vi "ConveyorBeltLoad.vi"(0 "Barcode":string) -> ()   [LabVIEW 2014]
uses:
  axxon_Gold.vi
panel:
  in  "Com2":T1
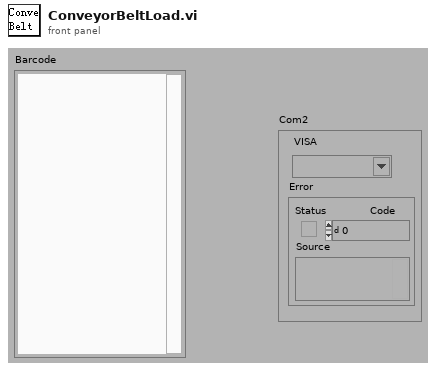
[diagram p1: front panel]
types:
  T1 = cluster{"VISA resource name out":refnum<visa-resource-name>, "error out":errorcluster}
  T2 = typedef "MoveSpeed.ctl" = cluster{"Speed of in board":dbl, "Acc of in board motor":dbl, "Stroke of in board motor":dbl, "Speed of adjusting width motor":dbl, "Acc of adjusting width motor":dbl, "Stroke of adjusting width motor":dbl, "Speed of motor running":dbl, "Acc of motor running":dbl, "Speed of out board":dbl, "Standby Motor Velocity":dbl, "Standby Motor Acceleration:":dbl, "Speed of reflowing motor":dbl, "Speed of reflowing Track Adjusting":dbl, "Acc of reflowing adjusting ":dbl, "Acc of reflowing motor":dbl, "Standby Motor delay":dbl}
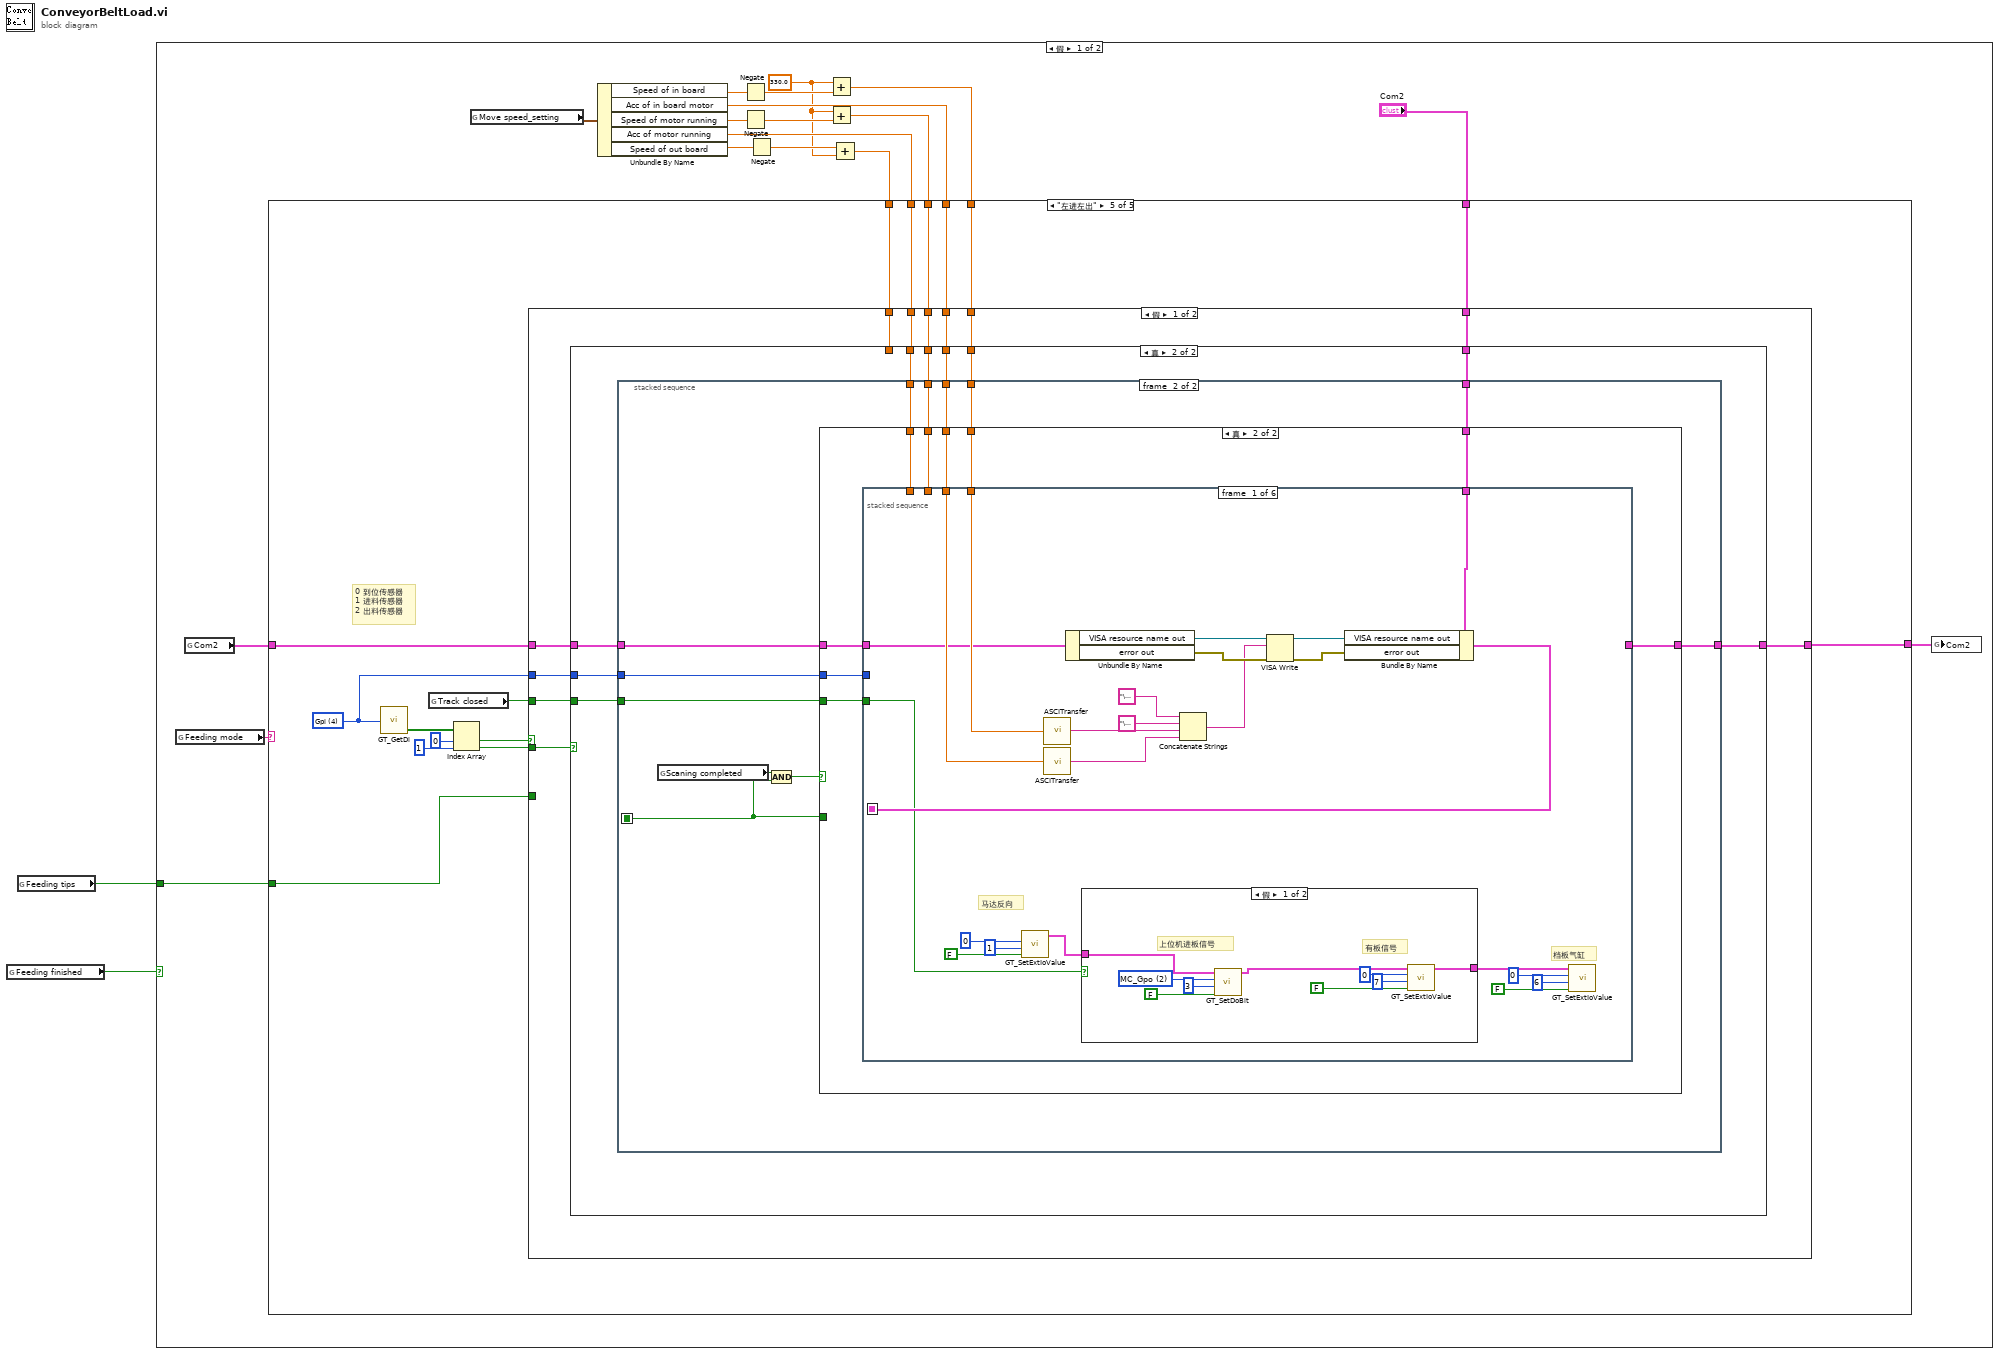
[diagram p0: block diagram]
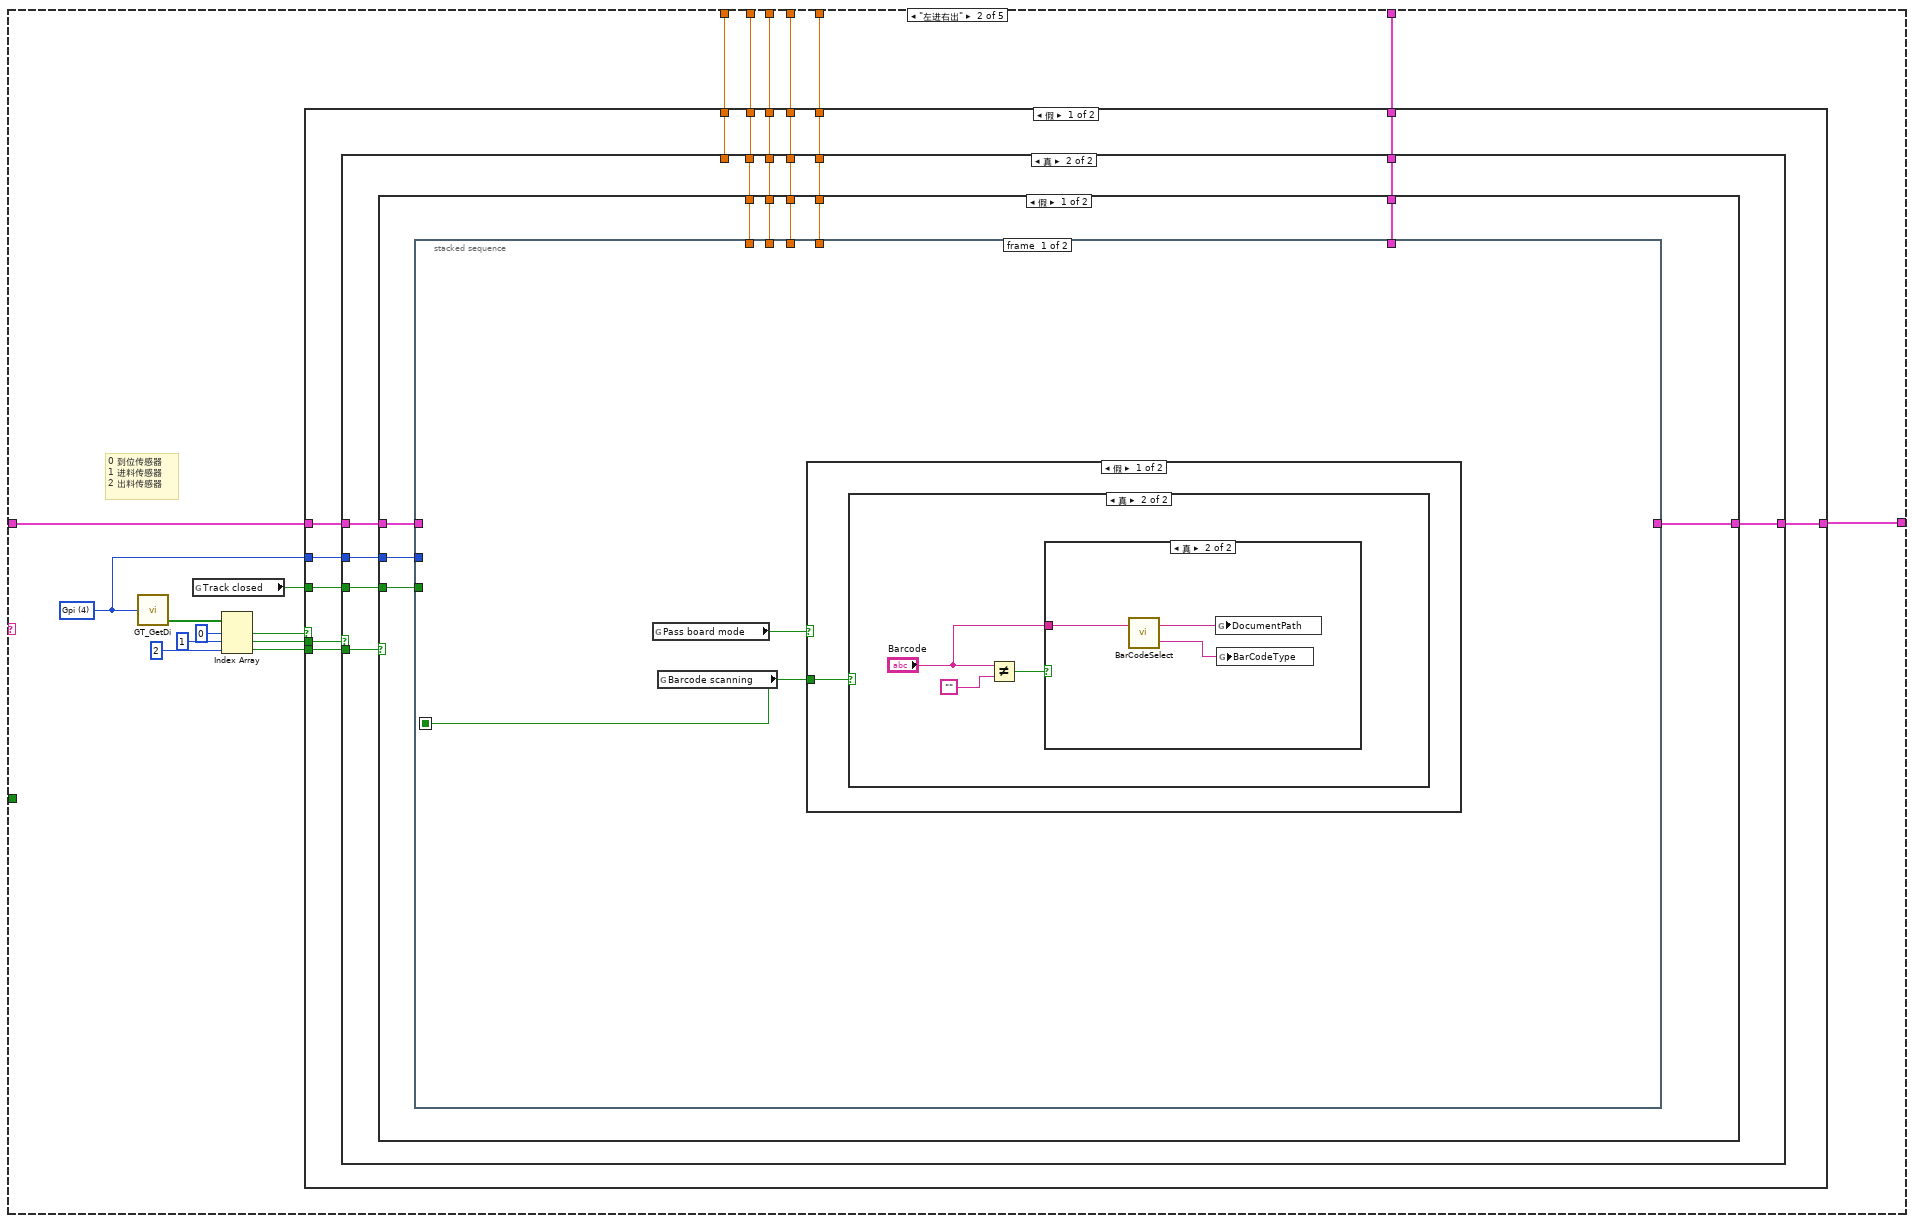
[diagram p3: hidden frame]
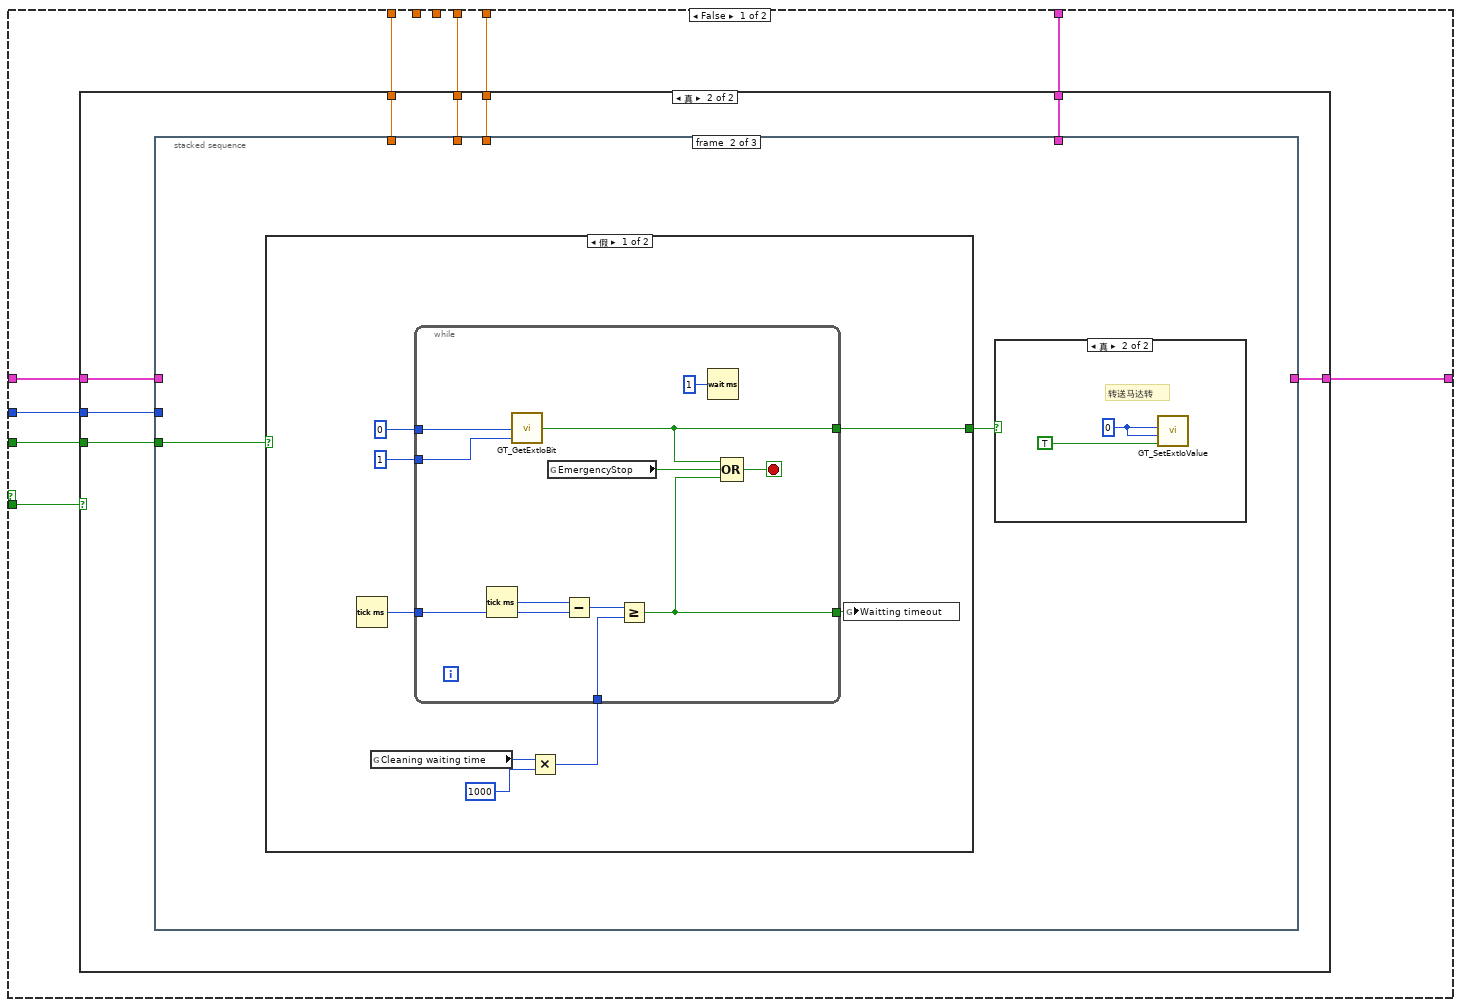
[diagram p4: hidden frame]
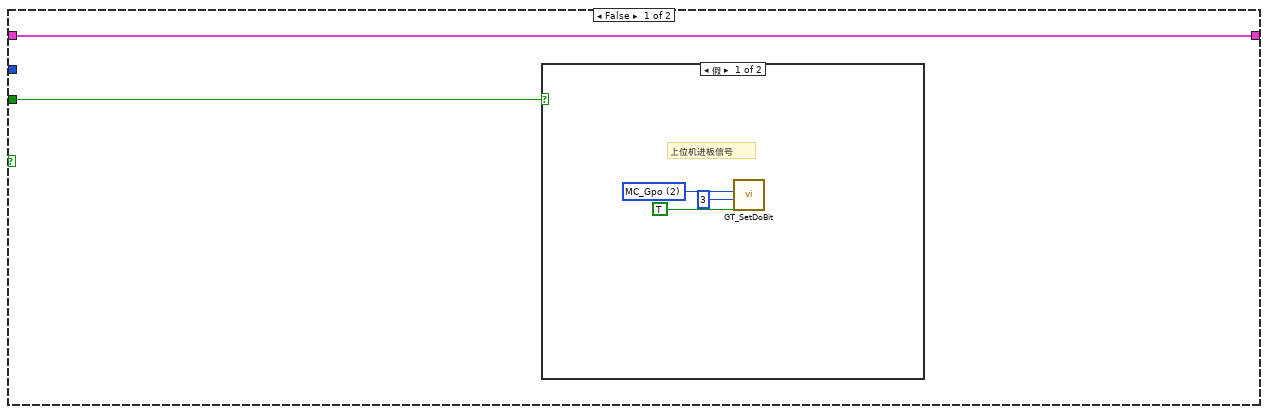
[diagram p5: hidden frame]
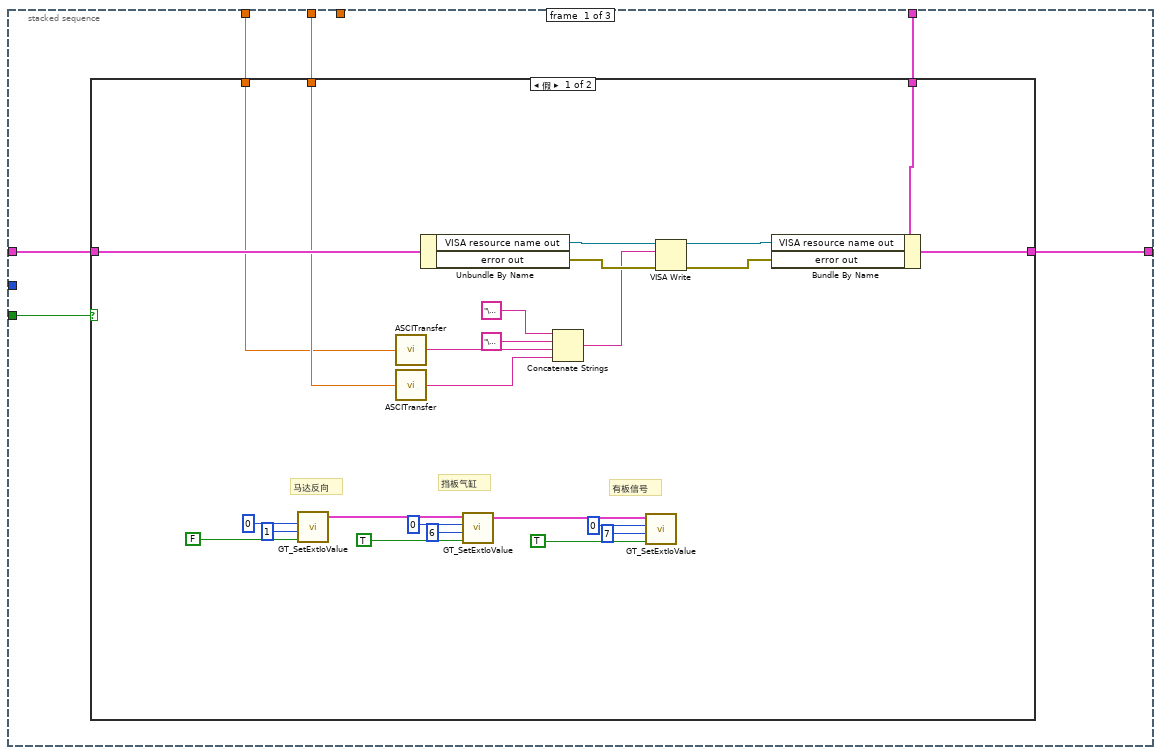
[diagram p7: hidden frame]
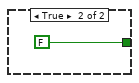
[diagram p10: hidden frame]
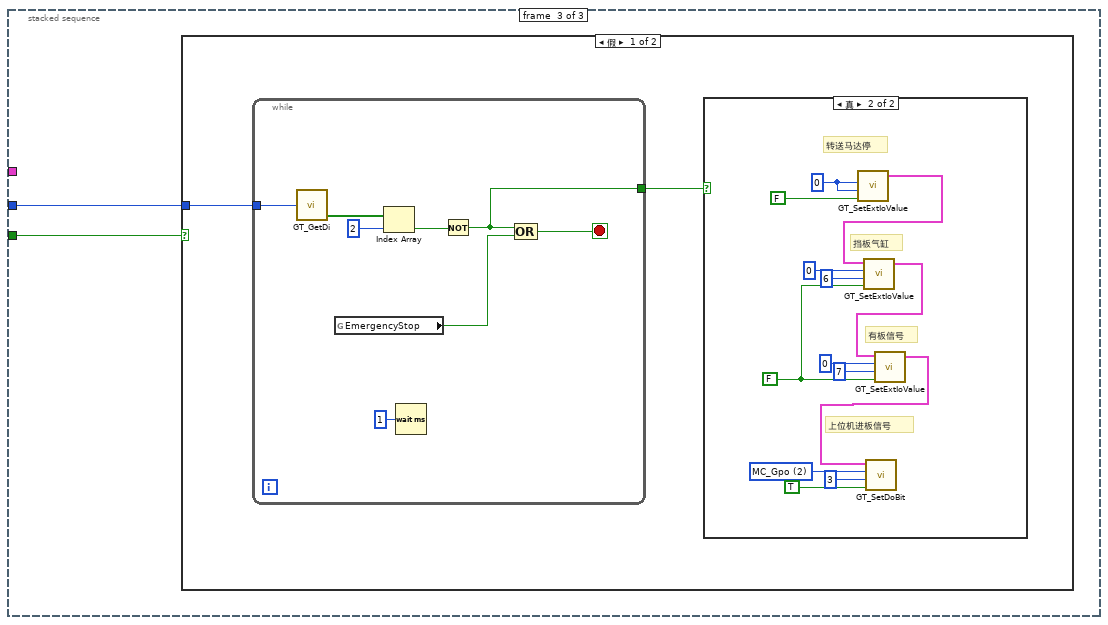
[diagram p11: hidden frame]
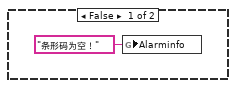
[diagram p15: hidden frame]
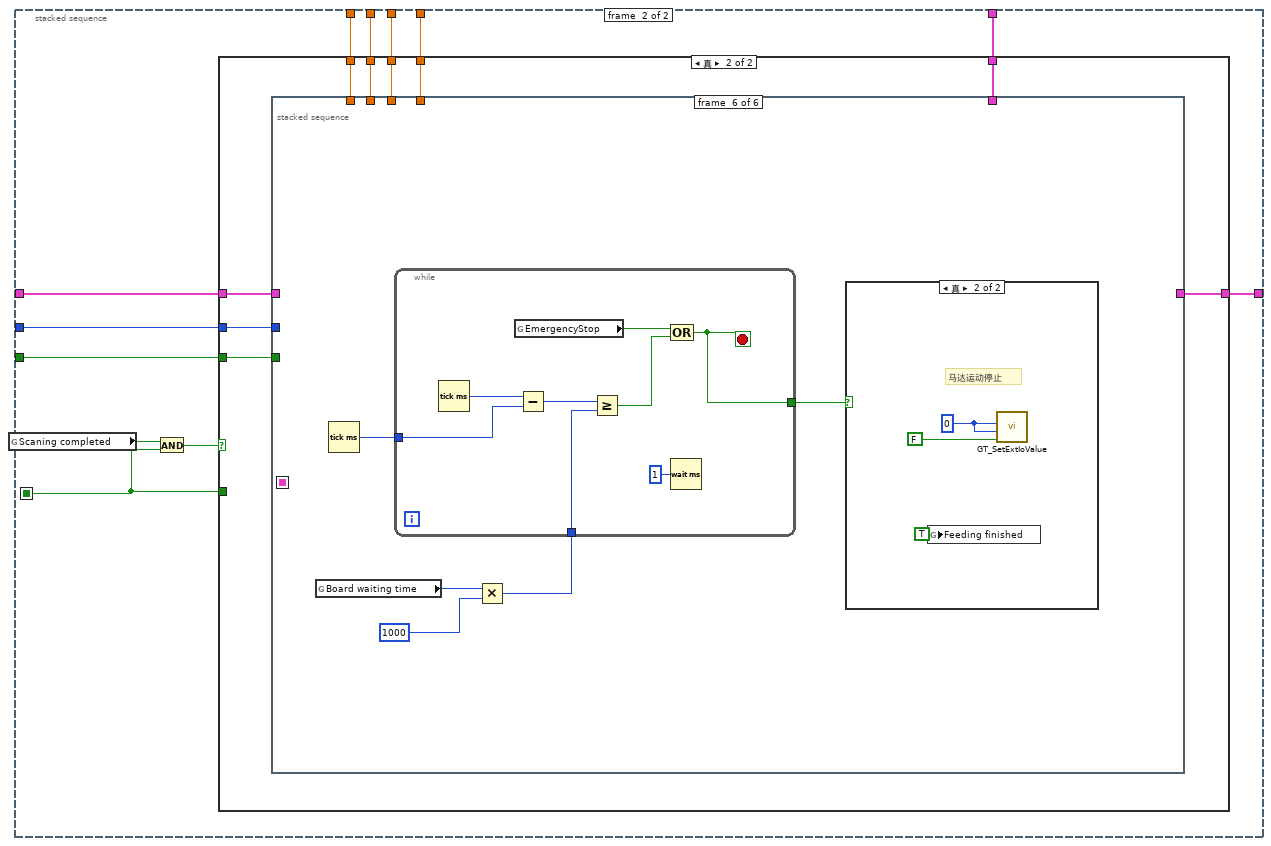
[diagram p17: hidden frame]
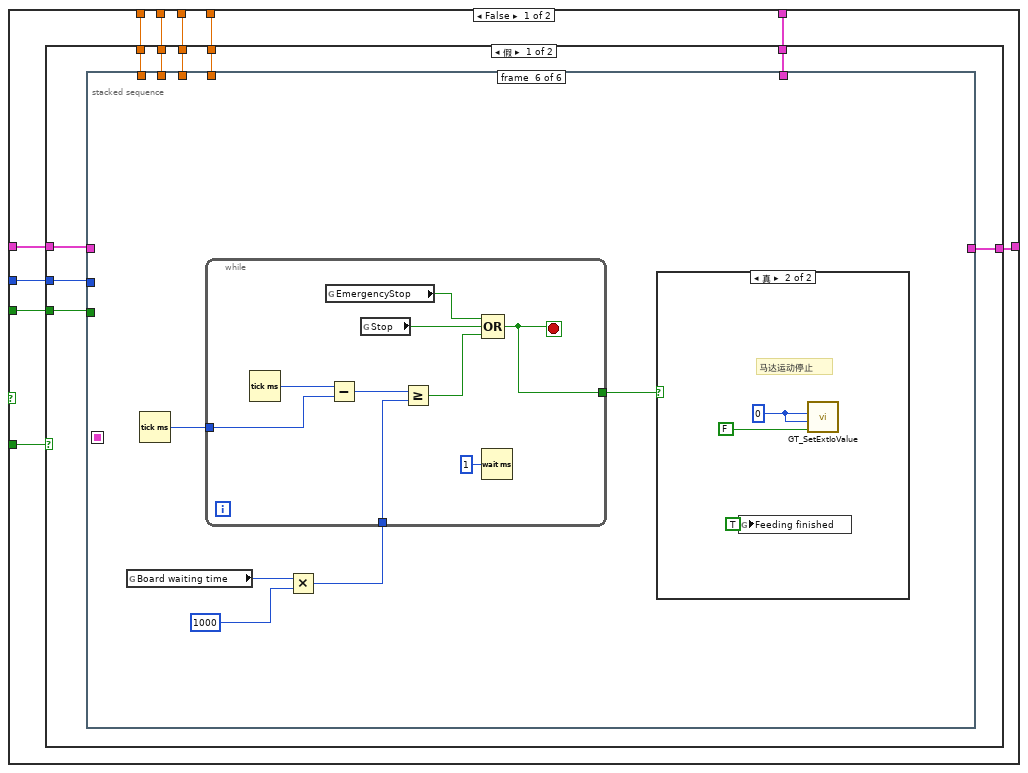
[diagram p18: hidden frame]
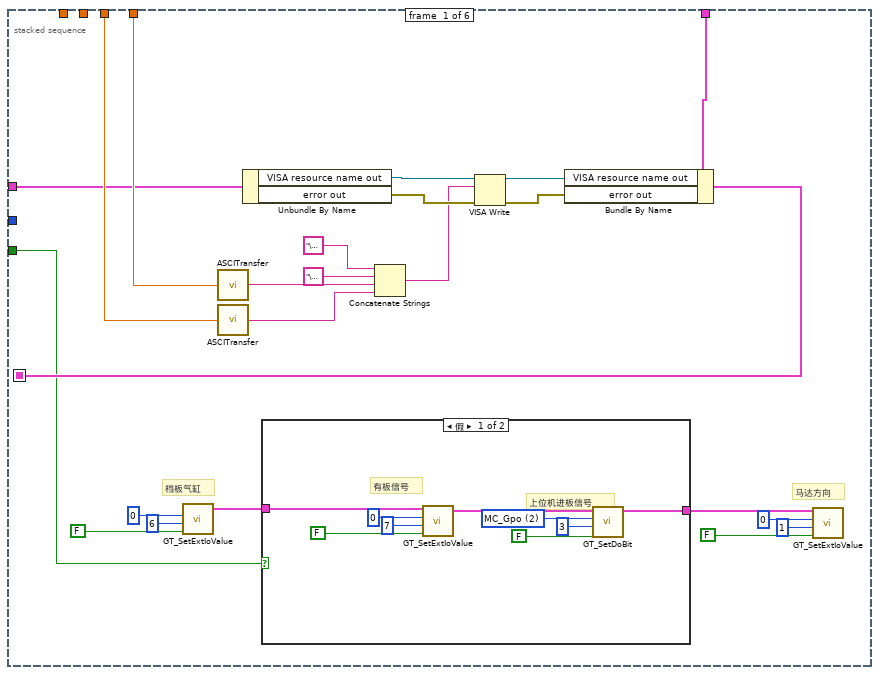
[diagram p19: hidden frame]
diagram:
  n1 = global read "axxon_Gold.vi" "Feeding finished"() -> (w2:bool)
  n2 = global read "axxon_Gold.vi" "Feeding tips"() -> (w1:bool)
  n3 = case shown="假" w2 {
    tunnel: w1 -> [w3 _]
    frame False {
      w7 = 330.0 ("x")
      n4 = global read "axxon_Gold.vi" "Feeding mode"() -> (w5:string)
      n5 = global read "axxon_Gold.vi" "Com2"() -> (w4:T1)
      n6 = global read "axxon_Gold.vi" "Move speed_setting"() -> (w20:T2)
      n7 = Unbundle By Name(w20) -> ("Speed of in board"=w19:dbl, "Acc of in board motor"=w18:dbl, "Speed of motor running"=w15:dbl, "Acc of motor running"=w14:dbl, "Speed of out board"=w9:dbl)
      n8 = Negate(x=w19) -> (-x=w13:dbl)
      n9 = Negate(x=w15) -> (-x=w11:dbl)
      n10 = Negate(x=w9) -> (-x=w8:dbl)
      n11 = Add(x=w7, y=w13) -> (x+y=w12:dbl)
      n12 = Add(x=w7, y=w11) -> (x+y=w10:dbl)
      n13 = Add(x=w8, y=w7) -> (x+y=w6:dbl)
      n14 = case shown="\"左进左出\"" w5 {
        tunnel: w18 -> [_ w31 w535 w1028 w1411]
        tunnel: "Com2" -> [_ w30 w534 w1027 w1410]
        tunnel: [w21 w29 w533 w1026 w1409] -> w16
        tunnel: w14 -> [_ w27 w531 w1024 w1407]
        tunnel: w12 -> [_ w25 w529 w1022 w1405]
        tunnel: w10 -> [_ w24 w528 w1021 w1404]
        tunnel: w6 -> [_ w23 w527 w1020 w1403]
        tunnel: w4 -> [w21 w22 w526 w1019 w1402]
        tunnel: w3 -> [_ _ _ w1018 w1401]
        frame Default {
        }
        frame "左进右出" {
          w28 = i16 4 items=["Limit_Positive", "Limit_Negative", "Alarm", "Home", "Gpi", "arrive"] ("diType in")
          # "0 到位传感器\n1 进料传感器\n2 出料传感器"
          n15 = call "GT_GetDi.vi"("diType in"=w28) -> ("IOOut"=w38:bool[])  [unwired: 2 in, 2 out]
          n16 = global read "axxon_Gold.vi" "Track closed"() -> (w26:bool)
          n17 = Index Array(array=w38, index #1=0 ("索引"), index #2=1 ("索引"), index #3=2 ("索引")) -> (element #1=w34:bool, element #2=w33:bool, element #3=w32:bool)
          n18 = case shown="假" w34 {
            tunnel: w33 -> [w50 _]
            tunnel: w32 -> [w49 _]
            tunnel: w25 -> [w48 w408]
            tunnel: w31 -> [w47 w407]
            tunnel: w30 -> [w46 w404]
            tunnel: w22 -> [w45 w406]
            tunnel: [w44 w405] -> w29
            tunnel: w28 -> [w43 w403]
            tunnel: w24 -> [w42 _]
            tunnel: w27 -> [w41 _]
            tunnel: w26 -> [w40 w402]
            tunnel: w23 -> [w39 w401]
            frame False {
              n19 = case shown="真" w50 {
                tunnel: w49 -> [w59 w163]
                tunnel: w48 -> [w55 w162]
                tunnel: w47 -> [w54 w161]
                tunnel: w46 -> [w56 w160]
                tunnel: w45 -> [w58 w159]
                tunnel: [w57 w158] -> w44
                tunnel: w43 -> [w53 w157]
                tunnel: w42 -> [_ w156]
                tunnel: w41 -> [_ w155]
                tunnel: w40 -> [w52 w154]
                tunnel: w39 -> [w51 _]
                frame False {
                  n20 = case shown="真" w59 {
                    tunnel: w58 -> [w61 w72]
                    tunnel: [w61 w71] -> w57
                    tunnel: w56 -> [_ w70]
                    tunnel: w55 -> [_ w69]
                    tunnel: w54 -> [_ w68]
                    tunnel: w53 -> [_ w67]
                    tunnel: w52 -> [w60 w66]
                    tunnel: w51 -> [_ w65]
                    frame False {
                      n21 = case shown="假" w60 {
                        frame False {
                          w64 = i16 2 items=["MC_Enable", "MC_Clear", "MC_Gpo"] ("doType")
                          # "上位机进板信号"
                          n22 = call "GT_SetDoBit.vi"("Value"=TRUE, "doIndex"=i16 3, "doType"=w64) -> ()  [unwired: 8 in, 1 out]
                        }
                        frame True {
                        }
                      }
                    }
                    frame True {
                      n23 = stacked-sequence {
                        tunnel: w72 -> [w78 _ _]
                        tunnel: [w77 _ _] -> w71
                        tunnel: w70 -> [w76 _ _]
                        tunnel: w69 -> [_ _ _]
                        tunnel: w68 -> [w75 _ _]
                        tunnel: w67 -> [_ _ w130]
                        tunnel: w66 -> [w73 w106 w129]
                        tunnel: w65 -> [w74 _ _]
                        frame #0 {
                          n24 = case shown="假" w73 {
                            tunnel: w78 -> [w94 w104]
                            tunnel: [w93 w104] -> w77
                            tunnel: w76 -> [w92 _]
                            tunnel: w75 -> [w91 _]
                            tunnel: w74 -> [w90 _]
                            frame False {
                              # "马达反向"
                              # "挡板气缸"
                              # "有板信号"
                              n25 = call "GT_SetExtIoValue.vi"("Value"=FALSE, "index"=1, "mdl"=0) -> ("rtn_Out"=w79:cluster{"rtn":i16, "Func":string})  [unwired: 3 in]
                              n26 = call "ASCITransfer.vi"("Input"=w90) -> ("Output"=w99:string)
                              n27 = call "ASCITransfer.vi"("Input"=w91) -> ("Output"=w98:string)
                              n28 = Unbundle By Name(w94) -> ("VISA resource name out"=w103:refnum<visa-resource-name>, "error out"=w102:errorcluster)
                              n29 = call "GT_SetExtIoValue.vi"("Value"=TRUE, "index"=6, "mdl"=0, "rtn_In"=w79) -> ("rtn_Out"=w83:cluster{"rtn":i16, "Func":string})  [unwired: 2 in]
                              n30 = Concatenate Strings("\u001f" ("字符串"), "\u0000" ("字符串"), w99, w98) -> (w97:string)
                              n31 = call "GT_SetExtIoValue.vi"("Value"=TRUE, "index"=7, "mdl"=0, "rtn_In"=w83) -> ()  [unwired: 2 in, 1 out]
                              n32 = VISA Write(VISA resource name=w103, write buffer=w97, error in (no error)=w102) -> (VISA resource name out=w96:refnum<visa-resource-name>, error out=w95:errorcluster)  [unwired: 1 out]
                              n33 = Bundle By Name(cluster=w92, "VISA resource name out"=w96, "error out"=w95) -> (w93:T1)
                            }
                            frame True {
                            }
                          }
                        }
                        frame #1 {
                          n34 = case shown="假" w106 {
                            tunnel: [w115 FALSE] -> w105
                            frame False {
                              n35 = Tick Count (ms)() -> (millisecond timer value=w111:u32)
                              n36 = global read "axxon_Gold.vi" "Cleaning waiting time"() -> (w113:i32)
                              n37 = Multiply(x=w113, y=1000) -> (x*y=w110:i32)
                              n38 = while {
                                tunnel: 0 ("mdl") -> [w127]
                                tunnel: [w122] -> w115
                                tunnel: 1 ("Index") -> [w124]
                                tunnel: w111 -> [w120]
                                tunnel: w110 -> [w118]
                                tunnel: [w117] -> w109
                                stop <- w125 stop-if-true
                                n39 = Tick Count (ms)() -> (millisecond timer value=w121:u32)
                                n40 = call "GT_GetExtIoBit.vi"("Index"=w124, "mdl"=w127) -> ("Status"=w122:bool)  [unwired: 2 in, 1 out]
                                n41 = global read "axxon_Gold.vi" "EmergencyStop"() -> (w123:bool)
                                n42 = Subtract(x=w121, y=w120) -> (x-y=w119:u32)
                                n43 = Greater Or Equal?(x=w119, y=w118) -> (x >= y?=w117:bool)
                                n44 = Wait (ms)(milliseconds to wait=u32 1 ("等待时间（毫秒）")) -> ()  [unwired: 1 out]
                                n45 = Compound Arithmetic op=OR(w122, w123, w117) -> (w125:bool)
                              }
                              n46 = global write "axxon_Gold.vi" "Waitting timeout"(w109) -> ()
                            }
                            frame True {
                            }
                          }
                          n47 = case shown="真" w105 {
                            frame False {
                            }
                            frame True {
                              w108 = 0 ("mdl")
                              # "转送马达转"
                              n48 = call "GT_SetExtIoValue.vi"("Value"=TRUE, "index"=w108, "mdl"=w108) -> ()  [unwired: 3 in, 1 out]
                            }
                          }
                        }
                        frame #2 {
                          n49 = case shown="假" w129 {
                            tunnel: w130 -> [w132 _]
                            frame False {
                              n50 = while {
                                tunnel: w132 -> [w153]
                                tunnel: [w146] -> w131
                                stop <- w148 stop-if-true
                                n51 = call "GT_GetDi.vi"("diType in"=w153) -> ("IOOut"=w152:bool[])  [unwired: 2 in, 2 out]
                                n52 = global read "axxon_Gold.vi" "EmergencyStop"() -> (w147:bool)
                                n53 = Index Array(array=w152, index=2 ("索引")) -> (element=w150:bool)
                                n54 = Wait (ms)(milliseconds to wait=u32 1 ("等待时间（毫秒）")) -> ()  [unwired: 1 out]
                                n55 = Not(x=w150) -> (.not. x?=w146:bool)
                                n56 = Compound Arithmetic op=OR(w146, w147) -> (w148:bool)
                              }
                              n57 = case shown="真" w131 {
                                frame False {
                                }
                                frame True {
                                w141 = i16 2 items=["MC_Enable", "MC_Clear", "MC_Gpo"] ("doType")
                                w134 = FALSE ("Value")
                                w145 = 0 ("mdl")
                                # "上位机进板信号"
                                # "有板信号"
                                # "挡板气缸"
                                # "转送马达停"
                                n58 = call "GT_SetExtIoValue.vi"("Value"=FALSE, "index"=w145, "mdl"=w145) -> ("rtn_Out"=w137:cluster{"rtn":i16, "Func":string})  [unwired: 3 in]
                                n59 = call "GT_SetExtIoValue.vi"("Value"=w134, "index"=6, "mdl"=0, "rtn_In"=w137) -> ("rtn_Out"=w133:cluster{"rtn":i16, "Func":string})  [unwired: 2 in]
                                n60 = call "GT_SetExtIoValue.vi"("Value"=w134, "index"=7, "mdl"=0, "rtn_In"=w133) -> ("rtn_Out"=w138:cluster{"rtn":i16, "Func":string})  [unwired: 2 in]
                                n61 = call "GT_SetDoBit.vi"("Value"=TRUE, "doIndex"=i16 3, "doType"=w141, "rtn_In"=w138) -> ()  [unwired: 7 in, 1 out]
                                }
                              }
                            }
                            frame True {
                            }
                          }
                        }
                      }
                    }
                  }
                }
                frame True {
                  n62 = case shown="假" w163 {
                    tunnel: w162 -> [w172 _]
                    tunnel: w161 -> [w171 _]
                    tunnel: w160 -> [w170 _]
                    tunnel: w159 -> [w169 w400]
                    tunnel: [w168 w400] -> w158
                    tunnel: w157 -> [w167 _]
                    tunnel: w156 -> [w166 _]
                    tunnel: w155 -> [w165 _]
                    tunnel: w154 -> [w164 _]
                    frame False {
                      n63 = stacked-sequence {
                        seq-local: [w173 _] -> [_ w183]
                        tunnel: w172 -> [_ w194]
                        tunnel: w171 -> [_ w193]
                        tunnel: w170 -> [_ w192]
                        tunnel: w169 -> [_ w191]
                        tunnel: [_ w190] -> w168
                        tunnel: w167 -> [_ w189]
                        tunnel: w166 -> [_ w188]
                        tunnel: w165 -> [_ w187]
                        tunnel: w164 -> [_ w186]
                        frame #0 {
                          n64 = global read "axxon_Gold.vi" "Pass board mode"() -> (w174:bool)
                          n65 = global read "axxon_Gold.vi" "Barcode scanning"() -> (w173:bool)
                          n66 = case shown="假" w174 {
                            tunnel: w173 -> [w175 _]
                            frame False {
                              n67 = case shown="真" w175 {
                                frame False {
                                }
                                frame True {
                                n68 = Not Equal?(x="Barcode", y="") -> (x != y?=w176:bool)
                                n69 = case shown="真" w176 {
                                tunnel: "Barcode" -> [_ w182]
                                frame False {
                                n70 = global write "axxon_Gold.vi" "Alarminfo"("条形码为空！" ("Alarminfo")) -> ()
                                }
                                frame True {
                                n71 = call "BarCodeSelect.vi"("BarcodeIn"=w182) -> ("ProductTyple"=w181:string, "ProgramPath"=w180:string)  [unwired: 1 in]
                                n72 = global write "axxon_Gold.vi" "DocumentPath"(w180) -> ()
                                n73 = global write "axxon_Gold.vi" "BarCodeType"(w181) -> ()
                                }
                                }
                                }
                              }
                            }
                            frame True {
                            }
                          }
                        }
                        frame #1 {
                          n74 = global read "axxon_Gold.vi" "Scaning completed"() -> (w184:bool)
                          n75 = And(x=w184, y=w183) -> (x .and. y?=w185:bool)
                          n76 = case shown="真" w185 {
                            tunnel: w194 -> [w197 w317]
                            tunnel: w193 -> [w198 w316]
                            tunnel: w192 -> [w196 w315]
                            tunnel: w191 -> [w203 w314]
                            tunnel: [w195 w313] -> w190
                            tunnel: w189 -> [w202 w312]
                            tunnel: w188 -> [w199 w311]
                            tunnel: w187 -> [w200 w310]
                            tunnel: w186 -> [w201 w309]
                            tunnel: w183 -> [w204 _]
                            frame False {
                              n77 = case shown="假" w204 {
                                tunnel: w203 -> [w213 w308]
                                tunnel: w202 -> [w212 _]
                                tunnel: w201 -> [w211 _]
                                tunnel: w200 -> [w210 _]
                                tunnel: w199 -> [w209 _]
                                tunnel: w198 -> [w208 _]
                                tunnel: w197 -> [w207 _]
                                tunnel: w196 -> [w206 _]
                                tunnel: [w205 w308] -> w195
                                frame False {
                                n78 = stacked-sequence {
                                seq-local: [w223 _ _ _ _ _] -> [_ _ _ w286 _ _]
                                tunnel: w207 -> [w232 _ _ _ _ _]
                                tunnel: w208 -> [w230 _ _ _ _ _]
                                tunnel: w206 -> [w227 _ _ w283 _ _]
                                tunnel: w213 -> [w224 _ _ _ _ _]
                                tunnel: [_ _ _ w282 _ _] -> w205
                                tunnel: w212 -> [_ _ w253 _ _ _]
                                tunnel: w209 -> [_ _ _ w277 _ _]
                                tunnel: w210 -> [_ _ _ w276 _ _]
                                tunnel: w211 -> [w222 _ _ _ _ _]
                                frame #0 {
                                # "马达方向"
                                # "档板气缸"
                                n79 = call "GT_SetExtIoValue.vi"("Value"=FALSE, "index"=6, "mdl"=0) -> ("rtn_Out"=w218:cluster{"rtn":i16, "Func":string})  [unwired: 3 in]
                                n80 = call "ASCITransfer.vi"("Input"=w232) -> ("Output"=w231:string)
                                n81 = call "ASCITransfer.vi"("Input"=w230) -> ("Output"=w229:string)
                                n82 = Unbundle By Name(w224) -> ("VISA resource name out"=w236:refnum<visa-resource-name>, "error out"=w235:errorcluster)
                                n83 = case shown="假" w222 {
                                tunnel: w218 -> [w242 w246]
                                tunnel: [w237 w246] -> w214
                                frame False {
                                w241 = i16 2 items=["MC_Enable", "MC_Clear", "MC_Gpo"] ("doType")
                                # "上位机进板信号"
                                # "有板信号"
                                n84 = call "GT_SetExtIoValue.vi"("Value"=FALSE, "index"=7, "mdl"=0, "rtn_In"=w242) -> ("rtn_Out"=w238:cluster{"rtn":i16, "Func":string})  [unwired: 2 in]
                                n85 = call "GT_SetDoBit.vi"("Value"=FALSE, "doIndex"=i16 3, "doType"=w241, "rtn_In"=w238) -> ("rtn_Out"=w237:cluster{"rtn":i16, "Func":string})  [unwired: 7 in]
                                }
                                frame True {
                                }
                                }
                                n86 = Concatenate Strings("\u001f" ("字符串"), "\u0000" ("字符串"), w231, w229) -> (w228:string)
                                n87 = VISA Write(VISA resource name=w236, write buffer=w228, error in (no error)=w235) -> (VISA resource name out=w226:refnum<visa-resource-name>, error out=w225:errorcluster)  [unwired: 1 out]
                                n88 = Bundle By Name(cluster=w227, "VISA resource name out"=w226, "error out"=w225) -> (w223:T1)
                                n89 = call "GT_SetExtIoValue.vi"("Value"=FALSE, "index"=1, "mdl"=0, "rtn_In"=w214) -> ()  [unwired: 2 in, 1 out]
                                }
                                frame #1 {
                                w249 = 0 ("mdl")
                                # "传送马达运动"
                                n90 = Wait (ms)(milliseconds to wait=u32 100 ("等待时间（毫秒）")) -> ()  [unwired: 1 out]
                                n91 = call "GT_SetExtIoValue.vi"("Value"=TRUE, "index"=w249, "mdl"=w249) -> ()  [unwired: 3 in, 1 out]
                                }
                                frame #2 {
                                n92 = Tick Count (ms)() -> (millisecond timer value=w251:u32)
                                n93 = while {
                                tunnel: w253 -> [w271]
                                tunnel: [w265] -> w252
                                tunnel: w251 -> [w263]
                                tunnel: u32 1500 ("y") -> [w261]
                                stop <- w265 stop-if-true
                                # "到位检测"
                                n94 = Tick Count (ms)() -> (millisecond timer value=w264:u32)
                                n95 = call "GT_GetDi.vi"("diType in"=w271) -> ("IOOut"=w270:bool[])  [unwired: 2 in, 2 out]
                                n96 = Wait (ms)(milliseconds to wait=u32 1 ("等待时间（毫秒）")) -> ()  [unwired: 1 out]
                                n97 = global read "axxon_Gold.vi" "EmergencyStop"() -> (w266:bool)
                                n98 = global read "axxon_Gold.vi" "Stop"() -> (w268:bool)
                                n99 = Subtract(x=w264, y=w263) -> (x-y=w262:u32)
                                n100 = Index Array(array=w270, index=0 ("索引")) -> (element=w260:bool)
                                n101 = Greater Or Equal?(x=w262, y=w261) -> (x >= y?=w259:bool)
                                n102 = case shown="假" w260 {
                                tunnel: w259 -> [w272 _]
                                frame False {
                                n103 = case shown="真" w272 {
                                frame False {
                                }
                                frame True {
                                w274 = 0 ("mdl")
                                n104 = call "GT_SetExtIoValue.vi"("Value"=TRUE, "index"=w274, "mdl"=w274) -> ()  [unwired: 3 in, 1 out]
                                }
                                }
                                }
                                frame True {
                                }
                                }
                                n105 = Compound Arithmetic op=OR(w260, w268, w266) -> (w265:bool)
                                }
                                n106 = case shown="真" w252 {
                                frame False {
                                }
                                frame True {
                                w254 = FALSE ("Value")
                                w258 = 0 ("mdl")
                                # "档板气缸"
                                # "传送马达停止"
                                n107 = call "GT_SetExtIoValue.vi"("Value"=w254, "index"=6, "mdl"=0) -> ("rtn_Out"=w255:cluster{"rtn":i16, "Func":string})  [unwired: 3 in]
                                n108 = call "GT_SetExtIoValue.vi"("Value"=w254, "index"=w258, "mdl"=w258, "rtn_In"=w255) -> ()  [unwired: 2 in, 1 out]
                                }
                                }
                                }
                                frame #3 {
                                n109 = call "ASCITransfer.vi"("Input"=w277) -> ("Output"=w279:string)
                                n110 = call "ASCITransfer.vi"("Input"=w276) -> ("Output"=w278:string)
                                n111 = Unbundle By Name(w286) -> ("VISA resource name out"=w288:refnum<visa-resource-name>, "error out"=w285:errorcluster)
                                n112 = Concatenate Strings("\u001f" ("字符串"), "\u0000" ("字符串"), w279, w278) -> (w275:string)
                                n113 = VISA Write(VISA resource name=w288, write buffer=w275, error in (no error)=w285) -> (VISA resource name out=w287:refnum<visa-resource-name>, error out=w284:errorcluster)  [unwired: 1 out]
                                n114 = Bundle By Name(cluster=w283, "VISA resource name out"=w287, "error out"=w284) -> (w282:T1)
                                }
                                frame #4 {
                                w290 = 0 ("mdl")
                                # "传送马达动"
                                n115 = call "GT_SetExtIoValue.vi"("Value"=TRUE, "index"=w290, "mdl"=w290) -> ()  [unwired: 3 in, 1 out]
                                }
                                frame #5 {
                                n116 = global read "axxon_Gold.vi" "Board waiting time"() -> (w294:u32)
                                n117 = Tick Count (ms)() -> (millisecond timer value=w295:u32)
                                n118 = Multiply(x=w294, y=u32 1000) -> (x*y=w292:u32)
                                n119 = while {
                                tunnel: w295 -> [w306]
                                tunnel: w292 -> [w304]
                                tunnel: [w300] -> w291
                                stop <- w300 stop-if-true
                                n120 = Tick Count (ms)() -> (millisecond timer value=w307:u32)
                                n121 = global read "axxon_Gold.vi" "EmergencyStop"() -> (w299:bool)
                                n122 = Subtract(x=w307, y=w306) -> (x-y=w305:u32)
                                n123 = global read "axxon_Gold.vi" "Stop"() -> (w303:bool)
                                n124 = Greater Or Equal?(x=w305, y=w304) -> (x >= y?=w302:bool)
                                n125 = Compound Arithmetic op=OR(w299, w303, w302) -> (w300:bool)
                                n126 = Wait (ms)(milliseconds to wait=u32 1 ("等待时间（毫秒）")) -> ()  [unwired: 1 out]
                                }
                                n127 = case shown="真" w291 {
                                frame False {
                                }
                                frame True {
                                w298 = 0 ("mdl")
                                # "马达运动停止"
                                n128 = global write "axxon_Gold.vi" "Feeding finished"(TRUE ("进板完成")) -> ()
                                n129 = call "GT_SetExtIoValue.vi"("Value"=FALSE, "index"=w298, "mdl"=w298) -> ()  [unwired: 3 in, 1 out]
                                }
                                }
                                }
                                }
                                }
                                frame True {
                                }
                              }
                            }
                            frame True {
                              n130 = stacked-sequence {
                                seq-local: [w327 _ _ _ _ _] -> [_ _ _ w379 _ _]
                                tunnel: w317 -> [w336 _ _ _ _ _]
                                tunnel: w316 -> [w334 _ _ _ _ _]
                                tunnel: w315 -> [w331 _ _ w376 _ _]
                                tunnel: w314 -> [w328 _ _ _ _ _]
                                tunnel: [_ _ _ w375 _ _] -> w313
                                tunnel: w312 -> [_ _ w354 _ _ _]
                                tunnel: w311 -> [_ _ _ w370 _ _]
                                tunnel: w310 -> [_ _ _ w369 _ _]
                                tunnel: w309 -> [w326 _ _ _ _ _]
                                frame #0 {
                                # "马达反向"
                                # "档板气缸"
                                n131 = call "GT_SetExtIoValue.vi"("Value"=FALSE, "index"=1, "mdl"=0) -> ("rtn_Out"=w318:cluster{"rtn":i16, "Func":string})  [unwired: 3 in]
                                n132 = call "ASCITransfer.vi"("Input"=w336) -> ("Output"=w335:string)
                                n133 = call "ASCITransfer.vi"("Input"=w334) -> ("Output"=w333:string)
                                n134 = Unbundle By Name(w328) -> ("VISA resource name out"=w340:refnum<visa-resource-name>, "error out"=w339:errorcluster)
                                n135 = case shown="假" w326 {
                                tunnel: w318 -> [w343 w350]
                                tunnel: [w341 w350] -> w322
                                frame False {
                                w349 = i16 2 items=["MC_Enable", "MC_Clear", "MC_Gpo"] ("doType")
                                # "有板信号"
                                # "上位机进板信号"
                                n136 = call "GT_SetDoBit.vi"("Value"=FALSE, "doIndex"=i16 3, "doType"=w349, "rtn_In"=w343) -> ("rtn_Out"=w342:cluster{"rtn":i16, "Func":string})  [unwired: 7 in]
                                n137 = call "GT_SetExtIoValue.vi"("Value"=FALSE, "index"=7, "mdl"=0, "rtn_In"=w342) -> ("rtn_Out"=w341:cluster{"rtn":i16, "Func":string})  [unwired: 2 in]
                                }
                                frame True {
                                }
                                }
                                n138 = Concatenate Strings("\u001f" ("字符串"), "\u0000" ("字符串"), w335, w333) -> (w332:string)
                                n139 = VISA Write(VISA resource name=w340, write buffer=w332, error in (no error)=w339) -> (VISA resource name out=w330:refnum<visa-resource-name>, error out=w329:errorcluster)  [unwired: 1 out]
                                n140 = Bundle By Name(cluster=w331, "VISA resource name out"=w330, "error out"=w329) -> (w327:T1)
                                n141 = call "GT_SetExtIoValue.vi"("Value"=FALSE, "index"=6, "mdl"=0, "rtn_In"=w322) -> ()  [unwired: 2 in, 1 out]
                                }
                                frame #1 {
                                w352 = 0 ("mdl")
                                # "传送马达运动"
                                n142 = call "GT_SetExtIoValue.vi"("Value"=TRUE, "index"=w352, "mdl"=w352) -> ()  [unwired: 3 in, 1 out]
                                }
                                frame #2 {
                                n143 = while {
                                tunnel: w354 -> [w367]
                                tunnel: [w362] -> w353
                                stop <- w362 stop-if-true
                                # "到位检测"
                                n144 = call "GT_GetDi.vi"("diType in"=w367) -> ("IOOut"=w366:bool[])  [unwired: 2 in, 2 out]
                                n145 = Wait (ms)(milliseconds to wait=u32 1 ("等待时间（毫秒）")) -> ()  [unwired: 1 out]
                                n146 = global read "axxon_Gold.vi" "EmergencyStop"() -> (w361:bool)
                                n147 = Index Array(array=w366, index=0 ("索引")) -> (element=w364:bool)
                                n148 = Compound Arithmetic op=OR(w364, w361) -> (w362:bool)
                                }
                                n149 = case shown="真" w353 {
                                frame False {
                                }
                                frame True {
                                w360 = 0 ("mdl")
                                # "档板气缸"
                                # "传送马达停止"
                                n150 = call "GT_SetExtIoValue.vi"("Value"=FALSE, "index"=6, "mdl"=0) -> ("rtn_Out"=w355:cluster{"rtn":i16, "Func":string})  [unwired: 3 in]
                                n151 = call "GT_SetExtIoValue.vi"("Value"=FALSE, "index"=w360, "mdl"=w360, "rtn_In"=w355) -> ()  [unwired: 2 in, 1 out]
                                }
                                }
                                }
                                frame #3 {
                                n152 = call "ASCITransfer.vi"("Input"=w370) -> ("Output"=w372:string)
                                n153 = call "ASCITransfer.vi"("Input"=w369) -> ("Output"=w371:string)
                                n154 = Unbundle By Name(w379) -> ("VISA resource name out"=w381:refnum<visa-resource-name>, "error out"=w378:errorcluster)
                                n155 = Concatenate Strings("\u001f" ("字符串"), "\u0000" ("字符串"), w372, w371) -> (w368:string)
                                n156 = VISA Write(VISA resource name=w381, write buffer=w368, error in (no error)=w378) -> (VISA resource name out=w380:refnum<visa-resource-name>, error out=w377:errorcluster)  [unwired: 1 out]
                                n157 = Bundle By Name(cluster=w376, "VISA resource name out"=w380, "error out"=w377) -> (w375:T1)
                                }
                                frame #4 {
                                w383 = 0 ("mdl")
                                # "传送马达动"
                                n158 = call "GT_SetExtIoValue.vi"("Value"=TRUE, "index"=w383, "mdl"=w383) -> ()  [unwired: 3 in, 1 out]
                                }
                                frame #5 {
                                n159 = global read "axxon_Gold.vi" "Board waiting time"() -> (w387:u32)
                                n160 = Tick Count (ms)() -> (millisecond timer value=w388:u32)
                                n161 = Multiply(x=w387, y=u32 1000) -> (x*y=w385:u32)
                                n162 = while {
                                tunnel: w388 -> [w398]
                                tunnel: w385 -> [w396]
                                tunnel: [w393] -> w384
                                stop <- w393 stop-if-true
                                n163 = Tick Count (ms)() -> (millisecond timer value=w399:u32)
                                n164 = global read "axxon_Gold.vi" "EmergencyStop"() -> (w392:bool)
                                n165 = Subtract(x=w399, y=w398) -> (x-y=w397:u32)
                                n166 = Greater Or Equal?(x=w397, y=w396) -> (x >= y?=w395:bool)
                                n167 = Compound Arithmetic op=OR(w392, w395) -> (w393:bool)
                                n168 = Wait (ms)(milliseconds to wait=u32 1 ("等待时间（毫秒）")) -> ()  [unwired: 1 out]
                                }
                                n169 = case shown="真" w384 {
                                frame False {
                                }
                                frame True {
                                w391 = 0 ("mdl")
                                # "马达运动停止"
                                n170 = global write "axxon_Gold.vi" "Feeding finished"(TRUE ("进板完成")) -> ()
                                n171 = call "GT_SetExtIoValue.vi"("Value"=FALSE, "index"=w391, "mdl"=w391) -> ()  [unwired: 3 in, 1 out]
                                }
                                }
                                }
                              }
                            }
                          }
                        }
                      }
                    }
                    frame True {
                    }
                  }
                }
              }
            }
            frame True {
              n172 = stacked-sequence {
                seq-local: [w412 _ _ _ _ _] -> [_ w434 w442 w445 w469 w497]
                tunnel: w408 -> [_ _ _ _ _ _]
                tunnel: w407 -> [w417 _ _ _ _ _]
                tunnel: w406 -> [w416 _ _ _ _ _]
                tunnel: [w415 _ _ _ _ _] -> w405
                tunnel: w404 -> [w414 _ _ _ _ _]
                tunnel: w403 -> [_ _ _ w447 _ w499]
                tunnel: w402 -> [_ _ _ w446 w470 w498]
                tunnel: w401 -> [w413 _ _ _ _ _]
                frame #0 {
                  n173 = Two Button Dialog(message="轨道上有板，是否继续涂！" ("消息"), 1:"取消" ("F按钮名称（“取消”）"), 2:"确定" ("T按钮名称（“确定”）")) -> (T button?=w412:bool)
                  n174 = case shown="真" w412 {
                    tunnel: w417 -> [w422 _]
                    tunnel: w416 -> [w421 w433]
                    tunnel: [w420 w433] -> w415
                    tunnel: w414 -> [w419 _]
                    tunnel: w413 -> [w418 _]
                    frame False {
                      n175 = call "ASCITransfer.vi"("Input"=w418) -> ("Output"=w427:string)
                      n176 = call "ASCITransfer.vi"("Input"=w422) -> ("Output"=w426:string)
                      n177 = Unbundle By Name(w421) -> ("VISA resource name out"=w431:refnum<visa-resource-name>, "error out"=w430:errorcluster)
                      n178 = Concatenate Strings("\u001f" ("字符串"), "\u0000" ("字符串"), w427, w426) -> (w425:string)
                      n179 = VISA Write(VISA resource name=w431, write buffer=w425, error in (no error)=w430) -> (VISA resource name out=w424:refnum<visa-resource-name>, error out=w423:errorcluster)  [unwired: 1 out]
                      n180 = Bundle By Name(cluster=w419, "VISA resource name out"=w424, "error out"=w423) -> (w420:T1)
                    }
                    frame True {
                      n181 = global write "axxon_Gold.vi" "Feeding finished"(TRUE ("进板完成")) -> ()
                    }
                  }
                }
                frame #1 {
                  n182 = case shown="假" w434 {
                    frame False {
                      # "马达反向"
                      # "挡板气缸"
                      n183 = call "GT_SetExtIoValue.vi"("Value"=TRUE, "index"=6, "mdl"=0) -> ("rtn_Out"=w435:cluster{"rtn":i16, "Func":string})  [unwired: 3 in]
                      n184 = call "GT_SetExtIoValue.vi"("Value"=FALSE, "index"=1, "mdl"=0, "rtn_In"=w435) -> ()  [unwired: 2 in, 1 out]
                    }
                    frame True {
                    }
                  }
                }
                frame #2 {
                  n185 = case shown="假" w442 {
                    frame False {
                      w444 = 0 ("mdl")
                      # "传送马达运动"
                      n186 = call "GT_SetExtIoValue.vi"("Value"=TRUE, "index"=w444, "mdl"=w444) -> ()  [unwired: 3 in, 1 out]
                    }
                    frame True {
                    }
                  }
                }
                frame #3 {
                  n187 = case shown="假" w445 {
                    tunnel: w447 -> [w450 _]
                    tunnel: w446 -> [w448 _]
                    frame False {
                      n188 = while {
                        tunnel: w450 -> [w468]
                        tunnel: [w463] -> w449
                        stop <- w463 stop-if-true
                        n189 = call "GT_GetDi.vi"("diType in"=w468) -> ("IOOut"=w467:bool[])  [unwired: 2 in, 2 out]
                        n190 = global read "axxon_Gold.vi" "EmergencyStop"() -> (w462:bool)
                        n191 = Index Array(array=w467, index=2 ("索引")) -> (element=w465:bool)
                        n192 = Compound Arithmetic op=OR(w465, w462) -> (w463:bool)
                        n193 = Wait (ms)(milliseconds to wait=u32 1 ("等待时间（毫秒）")) -> ()  [unwired: 1 out]
                      }
                      n194 = case shown="真" w449 {
                        tunnel: w448 -> [_ w451]
                        frame False {
                        }
                        frame True {
                          n195 = stacked-sequence {
                            tunnel: w451 -> [w452 _]
                            frame #0 {
                              n196 = case shown="真" w452 {
                                frame False {
                                }
                                frame True {
                                n197 = global read "axxon_Gold.vi" "Discharge waiting time"() -> (w455:dbl)
                                n198 = Multiply(x=w455, y=1000.0) -> (x*y=w453:dbl)
                                n199 = Wait (ms)(milliseconds to wait=w453) -> ()  [unwired: 1 out]
                                }
                              }
                            }
                            frame #1 {
                              w461 = 0 ("mdl")
                              # "挡板气缸"
                              # "传送马达停止"
                              n200 = call "GT_SetExtIoValue.vi"("Value"=FALSE, "index"=w461, "mdl"=w461) -> ("rtn_Out"=w456:cluster{"rtn":i16, "Func":string})  [unwired: 3 in]
                              n201 = call "GT_SetExtIoValue.vi"("Value"=FALSE, "index"=6, "mdl"=0, "rtn_In"=w456) -> ()  [unwired: 2 in, 1 out]
                            }
                          }
                        }
                      }
                    }
                    frame True {
                    }
                  }
                }
                frame #4 {
                  n202 = case shown="假" w469 {
                    tunnel: w470 -> [w474 _]
                    frame False {
                      n203 = case shown="假" w474 {
                        tunnel: 0 ("mdl") -> [w484 _]
                        tunnel: [w483 FALSE] -> w472
                        tunnel: 1 ("Index") -> [w482 _]
                        frame False {
                          n204 = global read "axxon_Gold.vi" "Cleaning waiting time"() -> (w481:i32)
                          n205 = Tick Count (ms)() -> (millisecond timer value=w479:u32)
                          n206 = Multiply(x=w481, y=1000) -> (x*y=w478:i32)
                          n207 = while {
                            tunnel: w484 -> [w495]
                            tunnel: [w490] -> w483
                            tunnel: w482 -> [w492]
                            tunnel: w479 -> [w488]
                            tunnel: w478 -> [w486]
                            tunnel: [w485] -> w477
                            stop <- w493 stop-if-true
                            # "下位机进板信号"
                            n208 = Tick Count (ms)() -> (millisecond timer value=w489:u32)
                            n209 = call "GT_GetExtIoBit.vi"("Index"=w492, "mdl"=w495) -> ("Status"=w490:bool)  [unwired: 2 in, 1 out]
                            n210 = global read "axxon_Gold.vi" "EmergencyStop"() -> (w491:bool)
                            n211 = Subtract(x=w489, y=w488) -> (x-y=w487:u32)
                            n212 = Greater Or Equal?(x=w487, y=w486) -> (x >= y?=w485:bool)
                            n213 = Compound Arithmetic op=OR(w490, w491, w485) -> (w493:bool)
                            n214 = Wait (ms)(milliseconds to wait=u32 1 ("等待时间（毫秒）")) -> ()  [unwired: 1 out]
                          }
                          n215 = global write "axxon_Gold.vi" "Waitting timeout"(w477) -> ()
                        }
                        frame True {
                          # "离线模式"
                        }
                      }
                      n216 = case shown="假" w472 {
                        frame False {
                        }
                        frame True {
                          w476 = 0 ("mdl")
                          # "传送马达动"
                          n217 = call "GT_SetExtIoValue.vi"("Value"=TRUE, "index"=w476, "mdl"=w476) -> ()  [unwired: 3 in, 1 out]
                        }
                      }
                    }
                    frame True {
                    }
                  }
                }
                frame #5 {
                  n218 = case shown="假" w497 {
                    tunnel: w499 -> [w501 _]
                    tunnel: w498 -> [w500 _]
                    frame False {
                      n219 = case shown="假" w500 {
                        tunnel: w501 -> [w503 _]
                        frame False {
                          n220 = while {
                            tunnel: w503 -> [w525]
                            tunnel: [w520] -> w502
                            stop <- w520 stop-if-true
                            n221 = call "GT_GetDi.vi"("diType in"=w525) -> ("IOOut"=w524:bool[])  [unwired: 2 in, 2 out]
                            n222 = global read "axxon_Gold.vi" "EmergencyStop"() -> (w518:bool)
                            n223 = Index Array(array=w524, index=2 ("索引")) -> (element=w522:bool)
                            n224 = Not(x=w522) -> (.not. x?=w521:bool)
                            n225 = Wait (ms)(milliseconds to wait=u32 1 ("等待时间（毫秒）")) -> ()  [unwired: 1 out]
                            n226 = Compound Arithmetic op=OR(w521, w518) -> (w520:bool)
                          }
                          n227 = case shown="真" w502 {
                            frame False {
                            }
                            frame True {
                              w510 = i16 2 items=["MC_Enable", "MC_Clear", "MC_Gpo"] ("doType")
                              w517 = 0 ("mdl")
                              # "上位机进板信号"
                              # "有板信号"
                              # "挡板气缸"
                              # "传送马达停"
                              n228 = call "GT_SetExtIoValue.vi"("Value"=FALSE, "index"=w517, "mdl"=w517) -> ("rtn_Out"=w506:cluster{"rtn":i16, "Func":string})  [unwired: 3 in]
                              n229 = call "GT_SetExtIoValue.vi"("Value"=FALSE, "index"=6, "mdl"=0, "rtn_In"=w506) -> ("rtn_Out"=w505:cluster{"rtn":i16, "Func":string})  [unwired: 2 in]
                              n230 = call "GT_SetExtIoValue.vi"("Value"=FALSE, "index"=7, "mdl"=0, "rtn_In"=w505) -> ("rtn_Out"=w504:cluster{"rtn":i16, "Func":string})  [unwired: 2 in]
                              n231 = call "GT_SetDoBit.vi"("Value"=TRUE, "doIndex"=i16 3, "doType"=w510, "rtn_In"=w504) -> ()  [unwired: 7 in, 1 out]
                            }
                          }
                        }
                        frame True {
                        }
                      }
                    }
                    frame True {
                    }
                  }
                }
              }
            }
          }
        }
        frame "右进左出" {
          w532 = i16 4 items=["Limit_Positive", "Limit_Negative", "Alarm", "Home", "Gpi", "arrive"] ("diType in")
          # "0 到位传感器\n1 出料传感器\n2 进料传感器"
          n232 = call "GT_GetDi.vi"("diType in"=w532) -> ("IOOut"=w542:bool[])  [unwired: 2 in, 2 out]
          n233 = global read "axxon_Gold.vi" "Track closed"() -> (w530:bool)
          n234 = Index Array(array=w542, index #1=0 ("索引"), index #2=2 ("索引"), index #3=1 ("索引")) -> (element #1=w538:bool, element #2=w537:bool, element #3=w536:bool)
          n235 = case shown="假" w538 {
            tunnel: w537 -> [w554 _]
            tunnel: w536 -> [w553 _]
            tunnel: w529 -> [w552 w901]
            tunnel: w535 -> [w551 w900]
            tunnel: w534 -> [w550 w897]
            tunnel: w526 -> [w549 w899]
            tunnel: [w548 w898] -> w533
            tunnel: w532 -> [w547 w896]
            tunnel: w528 -> [w546 _]
            tunnel: w531 -> [w545 _]
            tunnel: w530 -> [w544 w895]
            tunnel: w527 -> [w543 w894]
            frame False {
              n236 = case shown="真" w554 {
                tunnel: w553 -> [w563 w667]
                tunnel: w552 -> [w559 w666]
                tunnel: w551 -> [w558 w665]
                tunnel: w550 -> [w560 w664]
                tunnel: w549 -> [w562 w663]
                tunnel: [w561 w662] -> w548
                tunnel: w547 -> [w557 w661]
                tunnel: w546 -> [_ w660]
                tunnel: w545 -> [_ w659]
                tunnel: w544 -> [w556 w658]
                tunnel: w543 -> [w555 _]
                frame False {
                  n237 = case shown="真" w563 {
                    tunnel: w562 -> [w565 w576]
                    tunnel: [w565 w575] -> w561
                    tunnel: w560 -> [_ w574]
                    tunnel: w559 -> [_ w573]
                    tunnel: w558 -> [_ w572]
                    tunnel: w557 -> [_ w571]
                    tunnel: w556 -> [w564 w570]
                    tunnel: w555 -> [_ w569]
                    frame False {
                      n238 = case shown="真" w564 {
                        frame False {
                          w568 = i16 2 items=["MC_Enable", "MC_Clear", "MC_Gpo"] ("doType")
                          # "上位机进板信号"
                          n239 = call "GT_SetDoBit.vi"("Value"=TRUE, "doIndex"=i16 3, "doType"=w568) -> ()  [unwired: 8 in, 1 out]
                        }
                        frame True {
                        }
                      }
                    }
                    frame True {
                      n240 = stacked-sequence {
                        tunnel: w576 -> [w582 _ _]
                        tunnel: [w581 _ _] -> w575
                        tunnel: w574 -> [w580 _ _]
                        tunnel: w573 -> [_ _ _]
                        tunnel: w572 -> [w579 _ _]
                        tunnel: w571 -> [_ _ w634]
                        tunnel: w570 -> [w577 w610 w633]
                        tunnel: w569 -> [w578 _ _]
                        frame #0 {
                          n241 = case shown="真" w577 {
                            tunnel: w582 -> [w598 w608]
                            tunnel: [w597 w608] -> w581
                            tunnel: w580 -> [w596 _]
                            tunnel: w579 -> [w595 _]
                            tunnel: w578 -> [w594 _]
                            frame False {
                              # "马达反向"
                              # "挡板气缸"
                              # "有板信号"
                              n242 = call "ASCITransfer.vi"("Input"=w594) -> ("Output"=w603:string)
                              n243 = call "ASCITransfer.vi"("Input"=w595) -> ("Output"=w602:string)
                              n244 = call "GT_SetExtIoValue.vi"("Value"=TRUE, "index"=1, "mdl"=0) -> ("rtn_Out"=w583:cluster{"rtn":i16, "Func":string})  [unwired: 3 in]
                              n245 = Unbundle By Name(w598) -> ("VISA resource name out"=w607:refnum<visa-resource-name>, "error out"=w606:errorcluster)
                              n246 = Concatenate Strings("\u001f" ("字符串"), "\u0000" ("字符串"), w603, w602) -> (w601:string)
                              n247 = call "GT_SetExtIoValue.vi"("Value"=TRUE, "index"=6, "mdl"=0, "rtn_In"=w583) -> ("rtn_Out"=w587:cluster{"rtn":i16, "Func":string})  [unwired: 2 in]
                              n248 = VISA Write(VISA resource name=w607, write buffer=w601, error in (no error)=w606) -> (VISA resource name out=w600:refnum<visa-resource-name>, error out=w599:errorcluster)  [unwired: 1 out]
                              n249 = call "GT_SetExtIoValue.vi"("Value"=TRUE, "index"=7, "mdl"=0, "rtn_In"=w587) -> ()  [unwired: 2 in, 1 out]
                              n250 = Bundle By Name(cluster=w596, "VISA resource name out"=w600, "error out"=w599) -> (w597:T1)
                            }
                            frame True {
                            }
                          }
                        }
                        frame #1 {
                          n251 = case shown="假" w610 {
                            tunnel: [w619 FALSE] -> w609
                            frame False {
                              n252 = Tick Count (ms)() -> (millisecond timer value=w615:u32)
                              n253 = global read "axxon_Gold.vi" "Cleaning waiting time"() -> (w617:i32)
                              n254 = Multiply(x=w617, y=1000) -> (x*y=w614:i32)
                              n255 = while {
                                tunnel: 0 ("mdl") -> [w631]
                                tunnel: [w626] -> w619
                                tunnel: 1 ("Index") -> [w628]
                                tunnel: w615 -> [w624]
                                tunnel: w614 -> [w622]
                                tunnel: [w621] -> w613
                                stop <- w629 stop-if-true
                                n256 = Tick Count (ms)() -> (millisecond timer value=w625:u32)
                                n257 = call "GT_GetExtIoBit.vi"("Index"=w628, "mdl"=w631) -> ("Status"=w626:bool)  [unwired: 2 in, 1 out]
                                n258 = global read "axxon_Gold.vi" "EmergencyStop"() -> (w627:bool)
                                n259 = Subtract(x=w625, y=w624) -> (x-y=w623:u32)
                                n260 = Greater Or Equal?(x=w623, y=w622) -> (x >= y?=w621:bool)
                                n261 = Wait (ms)(milliseconds to wait=u32 1 ("等待时间（毫秒）")) -> ()  [unwired: 1 out]
                                n262 = Compound Arithmetic op=OR(w626, w627, w621) -> (w629:bool)
                              }
                              n263 = global write "axxon_Gold.vi" "Waitting timeout"(w613) -> ()
                            }
                            frame True {
                            }
                          }
                          n264 = case shown="真" w609 {
                            frame False {
                            }
                            frame True {
                              w612 = 0 ("mdl")
                              # "转送马达转"
                              n265 = call "GT_SetExtIoValue.vi"("Value"=TRUE, "index"=w612, "mdl"=w612) -> ()  [unwired: 3 in, 1 out]
                            }
                          }
                        }
                        frame #2 {
                          n266 = case shown="假" w633 {
                            tunnel: w634 -> [w636 _]
                            frame False {
                              n267 = while {
                                tunnel: w636 -> [w657]
                                tunnel: [w650] -> w635
                                stop <- w652 stop-if-true
                                n268 = call "GT_GetDi.vi"("diType in"=w657) -> ("IOOut"=w656:bool[])  [unwired: 2 in, 2 out]
                                n269 = global read "axxon_Gold.vi" "EmergencyStop"() -> (w651:bool)
                                n270 = Index Array(array=w656, index=1 ("索引")) -> (element=w654:bool)
                                n271 = Wait (ms)(milliseconds to wait=u32 1 ("等待时间（毫秒）")) -> ()  [unwired: 1 out]
                                n272 = Not(x=w654) -> (.not. x?=w650:bool)
                                n273 = Compound Arithmetic op=OR(w650, w651) -> (w652:bool)
                              }
                              n274 = case shown="真" w635 {
                                frame False {
                                }
                                frame True {
                                w645 = i16 2 items=["MC_Enable", "MC_Clear", "MC_Gpo"] ("doType")
                                w638 = FALSE ("Value")
                                w649 = 0 ("mdl")
                                # "上位机进板信号"
                                # "有板信号"
                                # "挡板气缸"
                                # "转送马达停"
                                n275 = call "GT_SetExtIoValue.vi"("Value"=FALSE, "index"=w649, "mdl"=w649) -> ("rtn_Out"=w641:cluster{"rtn":i16, "Func":string})  [unwired: 3 in]
                                n276 = call "GT_SetExtIoValue.vi"("Value"=w638, "index"=6, "mdl"=0, "rtn_In"=w641) -> ("rtn_Out"=w637:cluster{"rtn":i16, "Func":string})  [unwired: 2 in]
                                n277 = call "GT_SetExtIoValue.vi"("Value"=w638, "index"=7, "mdl"=0, "rtn_In"=w637) -> ("rtn_Out"=w642:cluster{"rtn":i16, "Func":string})  [unwired: 2 in]
                                n278 = call "GT_SetDoBit.vi"("Value"=TRUE, "doIndex"=i16 3, "doType"=w645, "rtn_In"=w642) -> ()  [unwired: 7 in, 1 out]
                                }
                              }
                            }
                            frame True {
                            }
                          }
                        }
                      }
                    }
                  }
                }
                frame True {
                  n279 = case shown="假" w667 {
                    tunnel: w666 -> [w676 _]
                    tunnel: w665 -> [w675 _]
                    tunnel: w664 -> [w674 _]
                    tunnel: w663 -> [w673 w893]
                    tunnel: [w672 w893] -> w662
                    tunnel: w661 -> [w671 _]
                    tunnel: w660 -> [w670 _]
                    tunnel: w659 -> [w669 _]
                    tunnel: w658 -> [w668 _]
                    frame False {
                      n280 = stacked-sequence {
                        seq-local: [w677 _] -> [_ w687]
                        tunnel: w676 -> [_ w698]
                        tunnel: w675 -> [_ w697]
                        tunnel: w674 -> [_ w696]
                        tunnel: w673 -> [_ w695]
                        tunnel: [_ w694] -> w672
                        tunnel: w671 -> [_ w693]
                        tunnel: w670 -> [_ w692]
                        tunnel: w669 -> [_ w691]
                        tunnel: w668 -> [_ w690]
                        frame #0 {
                          n281 = global read "axxon_Gold.vi" "Pass board mode"() -> (w678:bool)
                          n282 = global read "axxon_Gold.vi" "Barcode scanning"() -> (w677:bool)
                          n283 = case shown="假" w678 {
                            tunnel: w677 -> [w679 _]
                            frame False {
                              n284 = case shown="假" w679 {
                                frame False {
                                }
                                frame True {
                                n285 = local read "Barcode"() -> (w680:string)
                                n286 = Not Equal?(x=w680, y="") -> (x != y?=w681:bool)
                                n287 = case shown="真" w681 {
                                tunnel: w680 -> [_ w686]
                                frame False {
                                n288 = global write "axxon_Gold.vi" "Alarminfo"("条形码为空！" ("Alarminfo")) -> ()
                                }
                                frame True {
                                n289 = call "BarCodeSelect.vi"("BarcodeIn"=w686) -> ("ProductTyple"=w684:string, "ProgramPath"=w685:string)  [unwired: 1 in]
                                n290 = global write "axxon_Gold.vi" "DocumentPath"(w685) -> ()
                                n291 = global write "axxon_Gold.vi" "BarCodeType"(w684) -> ()
                                }
                                }
                                }
                              }
                            }
                            frame True {
                            }
                          }
                        }
                        frame #1 {
                          n292 = global read "axxon_Gold.vi" "Scaning completed"() -> (w688:bool)
                          n293 = And(x=w688, y=w687) -> (x .and. y?=w689:bool)
                          n294 = case shown="假" w689 {
                            tunnel: w698 -> [w701 w810]
                            tunnel: w697 -> [w702 w809]
                            tunnel: w696 -> [w700 w808]
                            tunnel: w695 -> [w707 w807]
                            tunnel: [w699 w806] -> w694
                            tunnel: w693 -> [w706 w805]
                            tunnel: w692 -> [w703 w804]
                            tunnel: w691 -> [w704 w803]
                            tunnel: w690 -> [w705 w802]
                            tunnel: w687 -> [w708 _]
                            frame False {
                              n295 = case shown="假" w708 {
                                tunnel: w707 -> [w717 w801]
                                tunnel: w706 -> [w716 _]
                                tunnel: w705 -> [w715 _]
                                tunnel: w704 -> [w714 _]
                                tunnel: w703 -> [w713 _]
                                tunnel: w702 -> [w712 _]
                                tunnel: w701 -> [w711 _]
                                tunnel: w700 -> [w710 _]
                                tunnel: [w709 w801] -> w699
                                frame False {
                                n296 = stacked-sequence {
                                seq-local: [w727 _ _ _ _ _] -> [_ _ _ w779 _ _]
                                tunnel: w711 -> [w736 _ _ _ _ _]
                                tunnel: w712 -> [w734 _ _ _ _ _]
                                tunnel: w710 -> [w731 _ _ w776 _ _]
                                tunnel: w717 -> [w728 _ _ _ _ _]
                                tunnel: [_ _ _ w775 _ _] -> w709
                                tunnel: w716 -> [_ _ w754 _ _ _]
                                tunnel: w713 -> [_ _ _ w770 _ _]
                                tunnel: w714 -> [_ _ _ w769 _ _]
                                tunnel: w715 -> [w726 _ _ _ _ _]
                                frame #0 {
                                # "马达反向"
                                # "档板气缸"
                                n297 = call "GT_SetExtIoValue.vi"("Value"=FALSE, "index"=6, "mdl"=0) -> ("rtn_Out"=w722:cluster{"rtn":i16, "Func":string})  [unwired: 3 in]
                                n298 = call "ASCITransfer.vi"("Input"=w736) -> ("Output"=w735:string)
                                n299 = call "ASCITransfer.vi"("Input"=w734) -> ("Output"=w733:string)
                                n300 = Unbundle By Name(w728) -> ("VISA resource name out"=w740:refnum<visa-resource-name>, "error out"=w739:errorcluster)
                                n301 = case shown="假" w726 {
                                tunnel: w722 -> [w746 w750]
                                tunnel: [w741 w750] -> w718
                                frame False {
                                w745 = i16 2 items=["MC_Enable", "MC_Clear", "MC_Gpo"] ("doType")
                                # "上位机进板信号"
                                # "有板信号"
                                n302 = call "GT_SetExtIoValue.vi"("Value"=FALSE, "index"=7, "mdl"=0, "rtn_In"=w746) -> ("rtn_Out"=w742:cluster{"rtn":i16, "Func":string})  [unwired: 2 in]
                                n303 = call "GT_SetDoBit.vi"("Value"=FALSE, "doIndex"=i16 3, "doType"=w745, "rtn_In"=w742) -> ("rtn_Out"=w741:cluster{"rtn":i16, "Func":string})  [unwired: 7 in]
                                }
                                frame True {
                                }
                                }
                                n304 = Concatenate Strings("\u001f" ("字符串"), "\u0000" ("字符串"), w735, w733) -> (w732:string)
                                n305 = VISA Write(VISA resource name=w740, write buffer=w732, error in (no error)=w739) -> (VISA resource name out=w730:refnum<visa-resource-name>, error out=w729:errorcluster)  [unwired: 1 out]
                                n306 = Bundle By Name(cluster=w731, "VISA resource name out"=w730, "error out"=w729) -> (w727:T1)
                                n307 = call "GT_SetExtIoValue.vi"("Value"=TRUE, "index"=1, "mdl"=0, "rtn_In"=w718) -> ()  [unwired: 2 in, 1 out]
                                }
                                frame #1 {
                                w752 = 0 ("mdl")
                                # "传送马达运动"
                                n308 = call "GT_SetExtIoValue.vi"("Value"=TRUE, "index"=w752, "mdl"=w752) -> ()  [unwired: 3 in, 1 out]
                                }
                                frame #2 {
                                n309 = while {
                                tunnel: w754 -> [w767]
                                tunnel: [w761] -> w753
                                stop <- w761 stop-if-true
                                # "到位检测"
                                n310 = call "GT_GetDi.vi"("diType in"=w767) -> ("IOOut"=w766:bool[])  [unwired: 2 in, 2 out]
                                n311 = Wait (ms)(milliseconds to wait=u32 1 ("等待时间（毫秒）")) -> ()  [unwired: 1 out]
                                n312 = global read "axxon_Gold.vi" "EmergencyStop"() -> (w760:bool)
                                n313 = Index Array(array=w766, index=0 ("索引")) -> (element=w764:bool)
                                n314 = global read "axxon_Gold.vi" "Stop"() -> (w763:bool)
                                n315 = Compound Arithmetic op=OR(w764, w763, w760) -> (w761:bool)
                                }
                                n316 = case shown="真" w753 {
                                frame False {
                                }
                                frame True {
                                w755 = FALSE ("Value")
                                w759 = 0 ("mdl")
                                # "档板气缸"
                                # "传送马达停止"
                                n317 = call "GT_SetExtIoValue.vi"("Value"=w755, "index"=6, "mdl"=0) -> ("rtn_Out"=w756:cluster{"rtn":i16, "Func":string})  [unwired: 3 in]
                                n318 = call "GT_SetExtIoValue.vi"("Value"=w755, "index"=w759, "mdl"=w759, "rtn_In"=w756) -> ()  [unwired: 2 in, 1 out]
                                }
                                }
                                }
                                frame #3 {
                                n319 = call "ASCITransfer.vi"("Input"=w770) -> ("Output"=w772:string)
                                n320 = call "ASCITransfer.vi"("Input"=w769) -> ("Output"=w771:string)
                                n321 = Unbundle By Name(w779) -> ("VISA resource name out"=w781:refnum<visa-resource-name>, "error out"=w778:errorcluster)
                                n322 = Concatenate Strings("\u001f" ("字符串"), "\u0000" ("字符串"), w772, w771) -> (w768:string)
                                n323 = VISA Write(VISA resource name=w781, write buffer=w768, error in (no error)=w778) -> (VISA resource name out=w780:refnum<visa-resource-name>, error out=w777:errorcluster)  [unwired: 1 out]
                                n324 = Bundle By Name(cluster=w776, "VISA resource name out"=w780, "error out"=w777) -> (w775:T1)
                                }
                                frame #4 {
                                w783 = 0 ("mdl")
                                # "传送马达动"
                                n325 = call "GT_SetExtIoValue.vi"("Value"=TRUE, "index"=w783, "mdl"=w783) -> ()  [unwired: 3 in, 1 out]
                                }
                                frame #5 {
                                n326 = global read "axxon_Gold.vi" "Board waiting time"() -> (w787:u32)
                                n327 = Tick Count (ms)() -> (millisecond timer value=w788:u32)
                                n328 = Multiply(x=w787, y=u32 1000) -> (x*y=w785:u32)
                                n329 = while {
                                tunnel: w788 -> [w799]
                                tunnel: w785 -> [w797]
                                tunnel: [w793] -> w784
                                stop <- w793 stop-if-true
                                n330 = Tick Count (ms)() -> (millisecond timer value=w800:u32)
                                n331 = global read "axxon_Gold.vi" "EmergencyStop"() -> (w792:bool)
                                n332 = Subtract(x=w800, y=w799) -> (x-y=w798:u32)
                                n333 = global read "axxon_Gold.vi" "Stop"() -> (w796:bool)
                                n334 = Greater Or Equal?(x=w798, y=w797) -> (x >= y?=w795:bool)
                                n335 = Compound Arithmetic op=OR(w792, w796, w795) -> (w793:bool)
                                n336 = Wait (ms)(milliseconds to wait=u32 1 ("等待时间（毫秒）")) -> ()  [unwired: 1 out]
                                }
                                n337 = case shown="真" w784 {
                                frame False {
                                }
                                frame True {
                                w791 = 0 ("mdl")
                                # "马达运动停止"
                                n338 = global write "axxon_Gold.vi" "Feeding finished"(TRUE ("进板完成")) -> ()
                                n339 = call "GT_SetExtIoValue.vi"("Value"=FALSE, "index"=w791, "mdl"=w791) -> ()  [unwired: 3 in, 1 out]
                                }
                                }
                                }
                                }
                                }
                                frame True {
                                }
                              }
                            }
                            frame True {
                              n340 = stacked-sequence {
                                seq-local: [w820 _ _ _ _ _] -> [_ _ _ w872 _ _]
                                tunnel: w810 -> [w829 _ _ _ _ _]
                                tunnel: w809 -> [w827 _ _ _ _ _]
                                tunnel: w808 -> [w824 _ _ w869 _ _]
                                tunnel: w807 -> [w821 _ _ _ _ _]
                                tunnel: [_ _ _ w868 _ _] -> w806
                                tunnel: w805 -> [_ _ w847 _ _ _]
                                tunnel: w804 -> [_ _ _ w863 _ _]
                                tunnel: w803 -> [_ _ _ w862 _ _]
                                tunnel: w802 -> [w819 _ _ _ _ _]
                                frame #0 {
                                # "马达反向"
                                # "档板气缸"
                                n341 = call "GT_SetExtIoValue.vi"("Value"=TRUE, "index"=1, "mdl"=0) -> ("rtn_Out"=w811:cluster{"rtn":i16, "Func":string})  [unwired: 3 in]
                                n342 = call "ASCITransfer.vi"("Input"=w829) -> ("Output"=w828:string)
                                n343 = call "ASCITransfer.vi"("Input"=w827) -> ("Output"=w826:string)
                                n344 = Unbundle By Name(w821) -> ("VISA resource name out"=w833:refnum<visa-resource-name>, "error out"=w832:errorcluster)
                                n345 = case shown="假" w819 {
                                tunnel: w811 -> [w836 w843]
                                tunnel: [w834 w843] -> w815
                                frame False {
                                w842 = i16 2 items=["MC_Enable", "MC_Clear", "MC_Gpo"] ("doType")
                                # "有板信号"
                                # "上位机进板信号"
                                n346 = call "GT_SetDoBit.vi"("Value"=FALSE, "doIndex"=i16 3, "doType"=w842, "rtn_In"=w836) -> ("rtn_Out"=w835:cluster{"rtn":i16, "Func":string})  [unwired: 7 in]
                                n347 = call "GT_SetExtIoValue.vi"("Value"=FALSE, "index"=7, "mdl"=0, "rtn_In"=w835) -> ("rtn_Out"=w834:cluster{"rtn":i16, "Func":string})  [unwired: 2 in]
                                }
                                frame True {
                                }
                                }
                                n348 = Concatenate Strings("\u001f" ("字符串"), "\u0000" ("字符串"), w828, w826) -> (w825:string)
                                n349 = VISA Write(VISA resource name=w833, write buffer=w825, error in (no error)=w832) -> (VISA resource name out=w823:refnum<visa-resource-name>, error out=w822:errorcluster)  [unwired: 1 out]
                                n350 = Bundle By Name(cluster=w824, "VISA resource name out"=w823, "error out"=w822) -> (w820:T1)
                                n351 = call "GT_SetExtIoValue.vi"("Value"=FALSE, "index"=6, "mdl"=0, "rtn_In"=w815) -> ()  [unwired: 2 in, 1 out]
                                }
                                frame #1 {
                                w845 = 0 ("mdl")
                                # "传送马达运动"
                                n352 = call "GT_SetExtIoValue.vi"("Value"=TRUE, "index"=w845, "mdl"=w845) -> ()  [unwired: 3 in, 1 out]
                                }
                                frame #2 {
                                n353 = while {
                                tunnel: w847 -> [w860]
                                tunnel: [w855] -> w846
                                stop <- w855 stop-if-true
                                # "到位检测"
                                n354 = call "GT_GetDi.vi"("diType in"=w860) -> ("IOOut"=w859:bool[])  [unwired: 2 in, 2 out]
                                n355 = Wait (ms)(milliseconds to wait=u32 1 ("等待时间（毫秒）")) -> ()  [unwired: 1 out]
                                n356 = global read "axxon_Gold.vi" "EmergencyStop"() -> (w854:bool)
                                n357 = Index Array(array=w859, index=0 ("索引")) -> (element=w857:bool)
                                n358 = Compound Arithmetic op=OR(w857, w854) -> (w855:bool)
                                }
                                n359 = case shown="真" w846 {
                                frame False {
                                }
                                frame True {
                                w853 = 0 ("mdl")
                                # "档板气缸"
                                # "传送马达停止"
                                n360 = call "GT_SetExtIoValue.vi"("Value"=FALSE, "index"=6, "mdl"=0) -> ("rtn_Out"=w848:cluster{"rtn":i16, "Func":string})  [unwired: 3 in]
                                n361 = call "GT_SetExtIoValue.vi"("Value"=FALSE, "index"=w853, "mdl"=w853, "rtn_In"=w848) -> ()  [unwired: 2 in, 1 out]
                                }
                                }
                                }
                                frame #3 {
                                n362 = call "ASCITransfer.vi"("Input"=w863) -> ("Output"=w865:string)
                                n363 = call "ASCITransfer.vi"("Input"=w862) -> ("Output"=w864:string)
                                n364 = Unbundle By Name(w872) -> ("VISA resource name out"=w874:refnum<visa-resource-name>, "error out"=w871:errorcluster)
                                n365 = Concatenate Strings("\u001f" ("字符串"), "\u0000" ("字符串"), w865, w864) -> (w861:string)
                                n366 = VISA Write(VISA resource name=w874, write buffer=w861, error in (no error)=w871) -> (VISA resource name out=w873:refnum<visa-resource-name>, error out=w870:errorcluster)  [unwired: 1 out]
                                n367 = Bundle By Name(cluster=w869, "VISA resource name out"=w873, "error out"=w870) -> (w868:T1)
                                }
                                frame #4 {
                                w876 = 0 ("mdl")
                                # "传送马达动"
                                n368 = call "GT_SetExtIoValue.vi"("Value"=TRUE, "index"=w876, "mdl"=w876) -> ()  [unwired: 3 in, 1 out]
                                }
                                frame #5 {
                                n369 = global read "axxon_Gold.vi" "Board waiting time"() -> (w880:u32)
                                n370 = Tick Count (ms)() -> (millisecond timer value=w881:u32)
                                n371 = Multiply(x=w880, y=u32 1000) -> (x*y=w878:u32)
                                n372 = while {
                                tunnel: w881 -> [w891]
                                tunnel: w878 -> [w889]
                                tunnel: [w886] -> w877
                                stop <- w886 stop-if-true
                                n373 = Tick Count (ms)() -> (millisecond timer value=w892:u32)
                                n374 = global read "axxon_Gold.vi" "EmergencyStop"() -> (w885:bool)
                                n375 = Subtract(x=w892, y=w891) -> (x-y=w890:u32)
                                n376 = Greater Or Equal?(x=w890, y=w889) -> (x >= y?=w888:bool)
                                n377 = Compound Arithmetic op=OR(w885, w888) -> (w886:bool)
                                n378 = Wait (ms)(milliseconds to wait=u32 1 ("等待时间（毫秒）")) -> ()  [unwired: 1 out]
                                }
                                n379 = case shown="真" w877 {
                                frame False {
                                }
                                frame True {
                                w884 = 0 ("mdl")
                                # "马达运动停止"
                                n380 = global write "axxon_Gold.vi" "Feeding finished"(TRUE ("进板完成")) -> ()
                                n381 = call "GT_SetExtIoValue.vi"("Value"=FALSE, "index"=w884, "mdl"=w884) -> ()  [unwired: 3 in, 1 out]
                                }
                                }
                                }
                              }
                            }
                          }
                        }
                      }
                    }
                    frame True {
                    }
                  }
                }
              }
            }
            frame True {
              n382 = stacked-sequence {
                seq-local: [w905 _ _ _ _ _] -> [_ w927 w934 w937 w961 w989]
                tunnel: w901 -> [_ _ _ _ _ _]
                tunnel: w900 -> [w910 _ _ _ _ _]
                tunnel: w899 -> [w909 _ _ _ _ _]
                tunnel: [w908 _ _ _ _ _] -> w898
                tunnel: w897 -> [w907 _ _ _ _ _]
                tunnel: w896 -> [_ _ _ w939 _ w991]
                tunnel: w895 -> [_ _ _ w938 w962 w990]
                tunnel: w894 -> [w906 _ _ _ _ _]
                frame #0 {
                  n383 = Two Button Dialog(message="轨道上有板，是否继续涂！" ("消息"), 1:"取消" ("F按钮名称（“取消”）"), 2:"确定" ("T按钮名称（“确定”）")) -> (T button?=w905:bool)
                  n384 = case shown="真" w905 {
                    tunnel: w910 -> [w915 _]
                    tunnel: w909 -> [w914 w926]
                    tunnel: [w913 w926] -> w908
                    tunnel: w907 -> [w912 _]
                    tunnel: w906 -> [w911 _]
                    frame False {
                      n385 = call "ASCITransfer.vi"("Input"=w911) -> ("Output"=w920:string)
                      n386 = call "ASCITransfer.vi"("Input"=w915) -> ("Output"=w919:string)
                      n387 = Unbundle By Name(w914) -> ("VISA resource name out"=w924:refnum<visa-resource-name>, "error out"=w923:errorcluster)
                      n388 = Concatenate Strings("\u001f" ("字符串"), "\u0000" ("字符串"), w920, w919) -> (w918:string)
                      n389 = VISA Write(VISA resource name=w924, write buffer=w918, error in (no error)=w923) -> (VISA resource name out=w917:refnum<visa-resource-name>, error out=w916:errorcluster)  [unwired: 1 out]
                      n390 = Bundle By Name(cluster=w912, "VISA resource name out"=w917, "error out"=w916) -> (w913:T1)
                    }
                    frame True {
                      n391 = global write "axxon_Gold.vi" "Feeding finished"(TRUE ("进板完成")) -> ()
                    }
                  }
                }
                frame #1 {
                  n392 = case shown="假" w927 {
                    frame False {
                      # "马达反向"
                      # "挡板气缸"
                      n393 = call "GT_SetExtIoValue.vi"("Value"=TRUE, "index"=1, "mdl"=0) -> ()  [unwired: 3 in, 1 out]
                      n394 = call "GT_SetExtIoValue.vi"("Value"=TRUE, "index"=6, "mdl"=0) -> ()  [unwired: 3 in, 1 out]
                    }
                    frame True {
                    }
                  }
                }
                frame #2 {
                  n395 = case shown="假" w934 {
                    frame False {
                      w936 = 0 ("mdl")
                      # "传送马达运动"
                      n396 = call "GT_SetExtIoValue.vi"("Value"=TRUE, "index"=w936, "mdl"=w936) -> ()  [unwired: 3 in, 1 out]
                    }
                    frame True {
                    }
                  }
                }
                frame #3 {
                  n397 = case shown="假" w937 {
                    tunnel: w939 -> [w942 _]
                    tunnel: w938 -> [w940 _]
                    frame False {
                      n398 = while {
                        tunnel: w942 -> [w960]
                        tunnel: [w955] -> w941
                        stop <- w955 stop-if-true
                        n399 = call "GT_GetDi.vi"("diType in"=w960) -> ("IOOut"=w959:bool[])  [unwired: 2 in, 2 out]
                        n400 = global read "axxon_Gold.vi" "EmergencyStop"() -> (w954:bool)
                        n401 = Index Array(array=w959, index=1 ("索引")) -> (element=w957:bool)
                        n402 = Compound Arithmetic op=OR(w957, w954) -> (w955:bool)
                        n403 = Wait (ms)(milliseconds to wait=u32 1 ("等待时间（毫秒）")) -> ()  [unwired: 1 out]
                      }
                      n404 = case shown="真" w941 {
                        tunnel: w940 -> [_ w943]
                        frame False {
                        }
                        frame True {
                          n405 = stacked-sequence {
                            tunnel: w943 -> [w944 _]
                            frame #0 {
                              n406 = case shown="真" w944 {
                                frame False {
                                }
                                frame True {
                                n407 = global read "axxon_Gold.vi" "Discharge waiting time"() -> (w947:dbl)
                                n408 = Multiply(x=w947, y=1000.0) -> (x*y=w945:dbl)
                                n409 = Wait (ms)(milliseconds to wait=w945) -> ()  [unwired: 1 out]
                                }
                              }
                            }
                            frame #1 {
                              w953 = 0 ("mdl")
                              # "挡板气缸"
                              # "传送马达停止"
                              n410 = call "GT_SetExtIoValue.vi"("Value"=FALSE, "index"=w953, "mdl"=w953) -> ("rtn_Out"=w948:cluster{"rtn":i16, "Func":string})  [unwired: 3 in]
                              n411 = call "GT_SetExtIoValue.vi"("Value"=FALSE, "index"=6, "mdl"=0, "rtn_In"=w948) -> ()  [unwired: 2 in, 1 out]
                            }
                          }
                        }
                      }
                    }
                    frame True {
                    }
                  }
                }
                frame #4 {
                  n412 = case shown="假" w961 {
                    tunnel: w962 -> [w966 _]
                    frame False {
                      n413 = case shown="假" w966 {
                        tunnel: 0 ("mdl") -> [w976 _]
                        tunnel: [w975 FALSE] -> w964
                        tunnel: 1 ("Index") -> [w974 _]
                        frame False {
                          n414 = global read "axxon_Gold.vi" "Cleaning waiting time"() -> (w973:i32)
                          n415 = Tick Count (ms)() -> (millisecond timer value=w971:u32)
                          n416 = Multiply(x=w973, y=1000) -> (x*y=w970:i32)
                          n417 = while {
                            tunnel: w976 -> [w987]
                            tunnel: [w982] -> w975
                            tunnel: w974 -> [w984]
                            tunnel: w971 -> [w980]
                            tunnel: w970 -> [w978]
                            tunnel: [w977] -> w969
                            stop <- w985 stop-if-true
                            # "下位机进板信号"
                            n418 = Tick Count (ms)() -> (millisecond timer value=w981:u32)
                            n419 = call "GT_GetExtIoBit.vi"("Index"=w984, "mdl"=w987) -> ("Status"=w982:bool)  [unwired: 2 in, 1 out]
                            n420 = global read "axxon_Gold.vi" "EmergencyStop"() -> (w983:bool)
                            n421 = Subtract(x=w981, y=w980) -> (x-y=w979:u32)
                            n422 = Greater Or Equal?(x=w979, y=w978) -> (x >= y?=w977:bool)
                            n423 = Compound Arithmetic op=OR(w982, w983, w977) -> (w985:bool)
                            n424 = Wait (ms)(milliseconds to wait=u32 1 ("等待时间（毫秒）")) -> ()  [unwired: 1 out]
                          }
                          n425 = global write "axxon_Gold.vi" "Waitting timeout"(w969) -> ()
                        }
                        frame True {
                          # "离线模式"
                        }
                      }
                      n426 = case shown="真" w964 {
                        frame False {
                        }
                        frame True {
                          w968 = 0 ("mdl")
                          # "传送马达动"
                          n427 = call "GT_SetExtIoValue.vi"("Value"=TRUE, "index"=w968, "mdl"=w968) -> ()  [unwired: 3 in, 1 out]
                        }
                      }
                    }
                    frame True {
                    }
                  }
                }
                frame #5 {
                  n428 = case shown="假" w989 {
                    tunnel: w991 -> [w993 _]
                    tunnel: w990 -> [w992 _]
                    frame False {
                      n429 = case shown="假" w992 {
                        tunnel: w993 -> [w995 _]
                        frame False {
                          n430 = while {
                            tunnel: w995 -> [w1017]
                            tunnel: [w1012] -> w994
                            stop <- w1012 stop-if-true
                            n431 = call "GT_GetDi.vi"("diType in"=w1017) -> ("IOOut"=w1016:bool[])  [unwired: 2 in, 2 out]
                            n432 = global read "axxon_Gold.vi" "EmergencyStop"() -> (w1010:bool)
                            n433 = Index Array(array=w1016, index=1 ("索引")) -> (element=w1014:bool)
                            n434 = Not(x=w1014) -> (.not. x?=w1013:bool)
                            n435 = Wait (ms)(milliseconds to wait=u32 1 ("等待时间（毫秒）")) -> ()  [unwired: 1 out]
                            n436 = Compound Arithmetic op=OR(w1013, w1010) -> (w1012:bool)
                          }
                          n437 = case shown="真" w994 {
                            frame False {
                            }
                            frame True {
                              w1002 = i16 2 items=["MC_Enable", "MC_Clear", "MC_Gpo"] ("doType")
                              w1009 = 0 ("mdl")
                              # "上位机进板信号"
                              # "有板信号"
                              # "挡板气缸"
                              # "传送马达停"
                              n438 = call "GT_SetExtIoValue.vi"("Value"=FALSE, "index"=w1009, "mdl"=w1009) -> ("rtn_Out"=w998:cluster{"rtn":i16, "Func":string})  [unwired: 3 in]
                              n439 = call "GT_SetExtIoValue.vi"("Value"=FALSE, "index"=6, "mdl"=0, "rtn_In"=w998) -> ("rtn_Out"=w997:cluster{"rtn":i16, "Func":string})  [unwired: 2 in]
                              n440 = call "GT_SetExtIoValue.vi"("Value"=FALSE, "index"=7, "mdl"=0, "rtn_In"=w997) -> ("rtn_Out"=w996:cluster{"rtn":i16, "Func":string})  [unwired: 2 in]
                              n441 = call "GT_SetDoBit.vi"("Value"=TRUE, "doIndex"=i16 3, "doType"=w1002, "rtn_In"=w996) -> ()  [unwired: 7 in, 1 out]
                            }
                          }
                        }
                        frame True {
                        }
                      }
                    }
                    frame True {
                    }
                  }
                }
              }
            }
          }
        }
        frame "右进右出" {
          w1025 = i16 4 items=["Limit_Positive", "Limit_Negative", "Alarm", "Home", "Gpi", "arrive"] ("diType in")
          # "0 到位传感器\n1 进料传感器\n2 出料传感器"
          n442 = call "GT_GetDi.vi"("diType in"=w1025) -> ("IOOut"=w1033:bool[])  [unwired: 2 in, 2 out]
          n443 = global read "axxon_Gold.vi" "Track closed"() -> (w1023:bool)
          n444 = Index Array(array=w1033, index #1=0 ("索引"), index #2=2 ("索引")) -> (element #1=w1030:bool, element #2=w1029:bool)
          n445 = case shown="假" w1030 {
            tunnel: w1029 -> [w1044 _]
            tunnel: w1022 -> [w1043 w1283]
            tunnel: w1028 -> [w1042 w1282]
            tunnel: w1027 -> [w1041 w1279]
            tunnel: w1019 -> [w1040 w1281]
            tunnel: [w1039 w1280] -> w1026
            tunnel: w1025 -> [w1038 w1278]
            tunnel: w1021 -> [w1037 _]
            tunnel: w1024 -> [w1036 _]
            tunnel: w1023 -> [w1035 w1277]
            tunnel: w1020 -> [w1034 w1276]
            tunnel: w1018 -> [_ w1275]
            frame False {
              n446 = case shown="真" w1044 {
                tunnel: w1043 -> [_ w1055]
                tunnel: w1042 -> [_ w1054]
                tunnel: w1041 -> [_ w1053]
                tunnel: w1040 -> [w1046 w1052]
                tunnel: [w1046 w1051] -> w1039
                tunnel: w1038 -> [_ w1050]
                tunnel: w1037 -> [_ w1049]
                tunnel: w1036 -> [_ w1048]
                tunnel: w1035 -> [_ w1047]
                tunnel: w1034 -> [_ _]
                frame False {
                  n447 = global write "axxon_Gold.vi" "Feeding tips"(FALSE ("进料提示")) -> ()
                }
                frame True {
                  n448 = stacked-sequence {
                    seq-local: [w1057 _] -> [_ w1067]
                    tunnel: w1055 -> [_ w1078]
                    tunnel: w1054 -> [_ w1077]
                    tunnel: w1053 -> [_ w1076]
                    tunnel: w1052 -> [_ w1075]
                    tunnel: [_ w1074] -> w1051
                    tunnel: w1050 -> [_ w1073]
                    tunnel: w1049 -> [_ w1072]
                    tunnel: w1048 -> [_ w1071]
                    tunnel: w1047 -> [_ w1070]
                    frame #0 {
                      n449 = global write "axxon_Gold.vi" "Feeding tips"(FALSE ("进料提示")) -> ()
                      n450 = global read "axxon_Gold.vi" "Pass board mode"() -> (w1058:bool)
                      n451 = global read "axxon_Gold.vi" "Barcode scanning"() -> (w1057:bool)
                      n452 = case shown="假" w1058 {
                        tunnel: w1057 -> [w1059 _]
                        frame False {
                          n453 = case shown="假" w1059 {
                            frame False {
                            }
                            frame True {
                              n454 = local read "Barcode"() -> (w1060:string)
                              n455 = Not Equal?(x=w1060, y="") -> (x != y?=w1061:bool)
                              n456 = case shown="真" w1061 {
                                tunnel: w1060 -> [_ w1066]
                                frame False {
                                n457 = global write "axxon_Gold.vi" "Alarminfo"("条形码为空！" ("Alarminfo")) -> ()
                                }
                                frame True {
                                n458 = call "BarCodeSelect.vi"("BarcodeIn"=w1066) -> ("ProductTyple"=w1064:string, "ProgramPath"=w1065:string)  [unwired: 1 in]
                                n459 = global write "axxon_Gold.vi" "DocumentPath"(w1065) -> ()
                                n460 = global write "axxon_Gold.vi" "BarCodeType"(w1064) -> ()
                                }
                              }
                            }
                          }
                        }
                        frame True {
                        }
                      }
                    }
                    frame #1 {
                      n461 = global read "axxon_Gold.vi" "Scaning completed"() -> (w1068:bool)
                      n462 = And(x=w1068, y=w1067) -> (x .and. y?=w1069:bool)
                      n463 = case shown="真" w1069 {
                        tunnel: w1078 -> [w1081 w1192]
                        tunnel: w1077 -> [w1082 w1191]
                        tunnel: w1076 -> [w1080 w1190]
                        tunnel: w1075 -> [w1087 w1189]
                        tunnel: [w1079 w1188] -> w1074
                        tunnel: w1073 -> [w1086 w1187]
                        tunnel: w1072 -> [w1083 w1186]
                        tunnel: w1071 -> [w1084 w1185]
                        tunnel: w1070 -> [w1085 w1184]
                        tunnel: w1067 -> [w1088 _]
                        frame False {
                          n464 = case shown="假" w1088 {
                            tunnel: w1087 -> [w1097 w1183]
                            tunnel: w1086 -> [w1096 _]
                            tunnel: w1085 -> [w1095 _]
                            tunnel: w1084 -> [w1094 _]
                            tunnel: w1083 -> [w1093 _]
                            tunnel: w1082 -> [w1092 _]
                            tunnel: w1081 -> [w1091 _]
                            tunnel: w1080 -> [w1090 _]
                            tunnel: [w1089 w1183] -> w1079
                            frame False {
                              n465 = stacked-sequence {
                                seq-local: [w1107 _ _ _ _ _ _ _] -> [_ _ _ _ w1160 _ _ _]
                                tunnel: w1091 -> [w1116 _ _ _ _ _ _ _]
                                tunnel: w1092 -> [w1114 _ _ _ _ _ _ _]
                                tunnel: w1090 -> [w1111 _ _ _ w1157 _ _ _]
                                tunnel: w1097 -> [w1108 _ _ _ _ _ _ _]
                                tunnel: [_ _ _ _ w1156 _ _ _] -> w1089
                                tunnel: w1096 -> [_ _ _ w1135 _ _ _ _]
                                tunnel: w1093 -> [_ _ _ _ w1151 _ _ _]
                                tunnel: w1094 -> [_ _ _ _ w1150 _ _ _]
                                tunnel: w1095 -> [w1106 _ _ _ _ _ _ _]
                                frame #0 {
                                # "马达反向"
                                # "档板气缸"
                                n466 = call "GT_SetExtIoValue.vi"("Value"=TRUE, "index"=1, "mdl"=0) -> ("rtn_Out"=w1098:cluster{"rtn":i16, "Func":string})  [unwired: 3 in]
                                n467 = call "ASCITransfer.vi"("Input"=w1116) -> ("Output"=w1115:string)
                                n468 = call "ASCITransfer.vi"("Input"=w1114) -> ("Output"=w1113:string)
                                n469 = Unbundle By Name(w1108) -> ("VISA resource name out"=w1120:refnum<visa-resource-name>, "error out"=w1119:errorcluster)
                                n470 = case shown="假" w1106 {
                                tunnel: w1098 -> [w1126 w1130]
                                tunnel: [w1121 w1130] -> w1102
                                frame False {
                                w1125 = i16 2 items=["MC_Enable", "MC_Clear", "MC_Gpo"] ("doType")
                                # "上位机进板信号"
                                # "有板信号"
                                n471 = call "GT_SetExtIoValue.vi"("Value"=FALSE, "index"=7, "mdl"=0, "rtn_In"=w1126) -> ("rtn_Out"=w1122:cluster{"rtn":i16, "Func":string})  [unwired: 2 in]
                                n472 = call "GT_SetDoBit.vi"("Value"=FALSE, "doIndex"=i16 3, "doType"=w1125, "rtn_In"=w1122) -> ("rtn_Out"=w1121:cluster{"rtn":i16, "Func":string})  [unwired: 7 in]
                                }
                                frame True {
                                }
                                }
                                n473 = Concatenate Strings("\u001f" ("字符串"), "\u0000" ("字符串"), w1115, w1113) -> (w1112:string)
                                n474 = VISA Write(VISA resource name=w1120, write buffer=w1112, error in (no error)=w1119) -> (VISA resource name out=w1110:refnum<visa-resource-name>, error out=w1109:errorcluster)  [unwired: 1 out]
                                n475 = Bundle By Name(cluster=w1111, "VISA resource name out"=w1110, "error out"=w1109) -> (w1107:T1)
                                n476 = call "GT_SetExtIoValue.vi"("Value"=FALSE, "index"=6, "mdl"=0, "rtn_In"=w1102) -> ()  [unwired: 2 in, 1 out]
                                }
                                frame #1 {
                                n477 = Wait (ms)(milliseconds to wait=u32 20 ("等待时间（毫秒）")) -> ()  [unwired: 1 out]
                                }
                                frame #2 {
                                w1132 = 0 ("mdl")
                                n478 = call "GT_SetExtIoValue.vi"("Value"=TRUE, "index"=w1132, "mdl"=w1132) -> ()  [unwired: 3 in, 1 out]
                                }
                                frame #3 {
                                n479 = while {
                                tunnel: w1135 -> [w1148]
                                tunnel: [w1142] -> w1134
                                stop <- w1142 stop-if-true
                                # "到位检测"
                                n480 = call "GT_GetDi.vi"("diType in"=w1148) -> ("IOOut"=w1147:bool[])  [unwired: 2 in, 2 out]
                                n481 = Wait (ms)(milliseconds to wait=u32 1 ("等待时间（毫秒）")) -> ()  [unwired: 1 out]
                                n482 = global read "axxon_Gold.vi" "EmergencyStop"() -> (w1141:bool)
                                n483 = Index Array(array=w1147, index=0 ("索引")) -> (element=w1145:bool)
                                n484 = global read "axxon_Gold.vi" "Stop"() -> (w1144:bool)
                                n485 = Compound Arithmetic op=OR(w1145, w1144, w1141) -> (w1142:bool)
                                }
                                n486 = case shown="真" w1134 {
                                frame False {
                                }
                                frame True {
                                w1136 = FALSE ("Value")
                                w1140 = 0 ("mdl")
                                # "档板气缸"
                                # "传送马达停止"
                                n487 = call "GT_SetExtIoValue.vi"("Value"=w1136, "index"=6, "mdl"=0) -> ("rtn_Out"=w1137:cluster{"rtn":i16, "Func":string})  [unwired: 3 in]
                                n488 = call "GT_SetExtIoValue.vi"("Value"=w1136, "index"=w1140, "mdl"=w1140, "rtn_In"=w1137) -> ()  [unwired: 2 in, 1 out]
                                }
                                }
                                }
                                frame #4 {
                                n489 = call "ASCITransfer.vi"("Input"=w1151) -> ("Output"=w1153:string)
                                n490 = call "ASCITransfer.vi"("Input"=w1150) -> ("Output"=w1152:string)
                                n491 = Unbundle By Name(w1160) -> ("VISA resource name out"=w1162:refnum<visa-resource-name>, "error out"=w1159:errorcluster)
                                n492 = Concatenate Strings("\u001f" ("字符串"), "\u0000" ("字符串"), w1153, w1152) -> (w1149:string)
                                n493 = VISA Write(VISA resource name=w1162, write buffer=w1149, error in (no error)=w1159) -> (VISA resource name out=w1161:refnum<visa-resource-name>, error out=w1158:errorcluster)  [unwired: 1 out]
                                n494 = Bundle By Name(cluster=w1157, "VISA resource name out"=w1161, "error out"=w1158) -> (w1156:T1)
                                }
                                frame #5 {
                                n495 = Wait (ms)(milliseconds to wait=u32 20 ("等待时间（毫秒）")) -> ()  [unwired: 1 out]
                                }
                                frame #6 {
                                w1165 = 0 ("mdl")
                                # "传送马达动"
                                n496 = call "GT_SetExtIoValue.vi"("Value"=TRUE, "index"=w1165, "mdl"=w1165) -> ()  [unwired: 3 in, 1 out]
                                }
                                frame #7 {
                                n497 = global read "axxon_Gold.vi" "Board waiting time"() -> (w1169:u32)
                                n498 = Tick Count (ms)() -> (millisecond timer value=w1170:u32)
                                n499 = Multiply(x=w1169, y=u32 1000) -> (x*y=w1167:u32)
                                n500 = while {
                                tunnel: w1170 -> [w1181]
                                tunnel: w1167 -> [w1179]
                                tunnel: [w1175] -> w1166
                                stop <- w1175 stop-if-true
                                n501 = Tick Count (ms)() -> (millisecond timer value=w1182:u32)
                                n502 = global read "axxon_Gold.vi" "EmergencyStop"() -> (w1174:bool)
                                n503 = Subtract(x=w1182, y=w1181) -> (x-y=w1180:u32)
                                n504 = global read "axxon_Gold.vi" "Stop"() -> (w1178:bool)
                                n505 = Greater Or Equal?(x=w1180, y=w1179) -> (x >= y?=w1177:bool)
                                n506 = Compound Arithmetic op=OR(w1174, w1178, w1177) -> (w1175:bool)
                                n507 = Wait (ms)(milliseconds to wait=u32 1 ("等待时间（毫秒）")) -> ()  [unwired: 1 out]
                                }
                                n508 = case shown="真" w1166 {
                                frame False {
                                }
                                frame True {
                                w1173 = 0 ("mdl")
                                # "马达运动停止"
                                n509 = global write "axxon_Gold.vi" "Feeding finished"(TRUE ("进板完成")) -> ()
                                n510 = call "GT_SetExtIoValue.vi"("Value"=FALSE, "index"=w1173, "mdl"=w1173) -> ()  [unwired: 3 in, 1 out]
                                }
                                }
                                }
                              }
                            }
                            frame True {
                            }
                          }
                        }
                        frame True {
                          n511 = stacked-sequence {
                            seq-local: [w1202 _ _ _ _ _] -> [_ _ _ w1254 _ _]
                            tunnel: w1192 -> [w1211 _ _ _ _ _]
                            tunnel: w1191 -> [w1209 _ _ _ _ _]
                            tunnel: w1190 -> [w1206 _ _ w1251 _ _]
                            tunnel: w1189 -> [w1203 _ _ _ _ _]
                            tunnel: [_ _ _ w1250 _ _] -> w1188
                            tunnel: w1187 -> [_ _ w1229 _ _ _]
                            tunnel: w1186 -> [_ _ _ w1245 _ _]
                            tunnel: w1185 -> [_ _ _ w1244 _ _]
                            tunnel: w1184 -> [w1201 _ _ _ _ _]
                            frame #0 {
                              # "马达反向"
                              # "档板气缸"
                              n512 = call "GT_SetExtIoValue.vi"("Value"=TRUE, "index"=1, "mdl"=0) -> ("rtn_Out"=w1193:cluster{"rtn":i16, "Func":string})  [unwired: 3 in]
                              n513 = call "ASCITransfer.vi"("Input"=w1211) -> ("Output"=w1210:string)
                              n514 = call "ASCITransfer.vi"("Input"=w1209) -> ("Output"=w1208:string)
                              n515 = Unbundle By Name(w1203) -> ("VISA resource name out"=w1215:refnum<visa-resource-name>, "error out"=w1214:errorcluster)
                              n516 = case shown="假" w1201 {
                                tunnel: w1193 -> [w1218 w1225]
                                tunnel: [w1216 w1225] -> w1197
                                frame False {
                                w1224 = i16 2 items=["MC_Enable", "MC_Clear", "MC_Gpo"] ("doType")
                                # "有板信号"
                                # "上位机进板信号"
                                n517 = call "GT_SetDoBit.vi"("Value"=FALSE, "doIndex"=i16 3, "doType"=w1224, "rtn_In"=w1218) -> ("rtn_Out"=w1217:cluster{"rtn":i16, "Func":string})  [unwired: 7 in]
                                n518 = call "GT_SetExtIoValue.vi"("Value"=FALSE, "index"=7, "mdl"=0, "rtn_In"=w1217) -> ("rtn_Out"=w1216:cluster{"rtn":i16, "Func":string})  [unwired: 2 in]
                                }
                                frame True {
                                }
                              }
                              n519 = Concatenate Strings("\u001f" ("字符串"), "\u0000" ("字符串"), w1210, w1208) -> (w1207:string)
                              n520 = VISA Write(VISA resource name=w1215, write buffer=w1207, error in (no error)=w1214) -> (VISA resource name out=w1205:refnum<visa-resource-name>, error out=w1204:errorcluster)  [unwired: 1 out]
                              n521 = Bundle By Name(cluster=w1206, "VISA resource name out"=w1205, "error out"=w1204) -> (w1202:T1)
                              n522 = call "GT_SetExtIoValue.vi"("Value"=FALSE, "index"=6, "mdl"=0, "rtn_In"=w1197) -> ()  [unwired: 2 in, 1 out]
                            }
                            frame #1 {
                              w1227 = 0 ("mdl")
                              # "传送马达运动"
                              n523 = call "GT_SetExtIoValue.vi"("Value"=TRUE, "index"=w1227, "mdl"=w1227) -> ()  [unwired: 3 in, 1 out]
                            }
                            frame #2 {
                              n524 = while {
                                tunnel: w1229 -> [w1242]
                                tunnel: [w1237] -> w1228
                                stop <- w1237 stop-if-true
                                # "到位检测"
                                n525 = call "GT_GetDi.vi"("diType in"=w1242) -> ("IOOut"=w1241:bool[])  [unwired: 2 in, 2 out]
                                n526 = Wait (ms)(milliseconds to wait=u32 1 ("等待时间（毫秒）")) -> ()  [unwired: 1 out]
                                n527 = global read "axxon_Gold.vi" "EmergencyStop"() -> (w1236:bool)
                                n528 = Index Array(array=w1241, index=0 ("索引")) -> (element=w1239:bool)
                                n529 = Compound Arithmetic op=OR(w1239, w1236) -> (w1237:bool)
                              }
                              n530 = case shown="真" w1228 {
                                frame False {
                                }
                                frame True {
                                w1235 = 0 ("mdl")
                                # "档板气缸"
                                # "传送马达停止"
                                n531 = call "GT_SetExtIoValue.vi"("Value"=FALSE, "index"=6, "mdl"=0) -> ("rtn_Out"=w1230:cluster{"rtn":i16, "Func":string})  [unwired: 3 in]
                                n532 = call "GT_SetExtIoValue.vi"("Value"=FALSE, "index"=w1235, "mdl"=w1235, "rtn_In"=w1230) -> ()  [unwired: 2 in, 1 out]
                                }
                              }
                            }
                            frame #3 {
                              n533 = call "ASCITransfer.vi"("Input"=w1245) -> ("Output"=w1247:string)
                              n534 = call "ASCITransfer.vi"("Input"=w1244) -> ("Output"=w1246:string)
                              n535 = Unbundle By Name(w1254) -> ("VISA resource name out"=w1256:refnum<visa-resource-name>, "error out"=w1253:errorcluster)
                              n536 = Concatenate Strings("\u001f" ("字符串"), "\u0000" ("字符串"), w1247, w1246) -> (w1243:string)
                              n537 = VISA Write(VISA resource name=w1256, write buffer=w1243, error in (no error)=w1253) -> (VISA resource name out=w1255:refnum<visa-resource-name>, error out=w1252:errorcluster)  [unwired: 1 out]
                              n538 = Bundle By Name(cluster=w1251, "VISA resource name out"=w1255, "error out"=w1252) -> (w1250:T1)
                            }
                            frame #4 {
                              w1258 = 0 ("mdl")
                              # "传送马达动"
                              n539 = call "GT_SetExtIoValue.vi"("Value"=TRUE, "index"=w1258, "mdl"=w1258) -> ()  [unwired: 3 in, 1 out]
                            }
                            frame #5 {
                              n540 = global read "axxon_Gold.vi" "Board waiting time"() -> (w1262:u32)
                              n541 = Tick Count (ms)() -> (millisecond timer value=w1263:u32)
                              n542 = Multiply(x=w1262, y=u32 1000) -> (x*y=w1260:u32)
                              n543 = while {
                                tunnel: w1263 -> [w1273]
                                tunnel: w1260 -> [w1271]
                                tunnel: [w1268] -> w1259
                                stop <- w1268 stop-if-true
                                n544 = Tick Count (ms)() -> (millisecond timer value=w1274:u32)
                                n545 = global read "axxon_Gold.vi" "EmergencyStop"() -> (w1267:bool)
                                n546 = Subtract(x=w1274, y=w1273) -> (x-y=w1272:u32)
                                n547 = Greater Or Equal?(x=w1272, y=w1271) -> (x >= y?=w1270:bool)
                                n548 = Compound Arithmetic op=OR(w1267, w1270) -> (w1268:bool)
                                n549 = Wait (ms)(milliseconds to wait=u32 1 ("等待时间（毫秒）")) -> ()  [unwired: 1 out]
                              }
                              n550 = case shown="真" w1259 {
                                frame False {
                                }
                                frame True {
                                w1266 = 0 ("mdl")
                                # "马达运动停止"
                                n551 = global write "axxon_Gold.vi" "Feeding finished"(TRUE ("进板完成")) -> ()
                                n552 = call "GT_SetExtIoValue.vi"("Value"=FALSE, "index"=w1266, "mdl"=w1266) -> ()  [unwired: 3 in, 1 out]
                                }
                              }
                            }
                          }
                        }
                      }
                    }
                  }
                }
              }
            }
            frame True {
              n553 = stacked-sequence {
                seq-local: [w1285 _ _ _ _ _] -> [_ w1313 w1317 w1320 w1344 w1372]
                tunnel: w1283 -> [_ _ _ _ _ _]
                tunnel: w1282 -> [w1290 _ _ _ _ _]
                tunnel: w1281 -> [w1289 _ _ _ _ _]
                tunnel: [w1288 _ _ _ _ _] -> w1280
                tunnel: w1279 -> [w1287 _ _ _ _ _]
                tunnel: w1278 -> [_ _ _ w1322 _ w1374]
                tunnel: w1277 -> [_ _ _ w1321 w1345 w1373]
                tunnel: w1276 -> [w1286 _ _ _ _ _]
                tunnel: w1275 -> [w1284 _ _ _ _ _]
                frame #0 {
                  n554 = case shown="真" w1284 {
                    tunnel: [TRUE ("T button?") w1296] -> w1285
                    frame False {
                    }
                    frame True {
                      n555 = global write "axxon_Gold.vi" "Feeding tips"(FALSE ("进料提示")) -> ()
                      n556 = Two Button Dialog(message="轨道上有板，是否继续涂！" ("消息"), 1:"取消" ("F按钮名称（“取消”）"), 2:"确定" ("T按钮名称（“确定”）")) -> (T button?=w1296:bool)
                    }
                  }
                  n557 = case shown="真" w1285 {
                    tunnel: w1290 -> [w1301 _]
                    tunnel: w1289 -> [w1300 w1312]
                    tunnel: [w1299 w1312] -> w1288
                    tunnel: w1287 -> [w1298 _]
                    tunnel: w1286 -> [w1297 _]
                    frame False {
                      n558 = call "ASCITransfer.vi"("Input"=w1297) -> ("Output"=w1306:string)
                      n559 = call "ASCITransfer.vi"("Input"=w1301) -> ("Output"=w1305:string)
                      n560 = Unbundle By Name(w1300) -> ("VISA resource name out"=w1310:refnum<visa-resource-name>, "error out"=w1309:errorcluster)
                      n561 = Concatenate Strings("\u001f" ("字符串"), "\u0000" ("字符串"), w1306, w1305) -> (w1304:string)
                      n562 = VISA Write(VISA resource name=w1310, write buffer=w1304, error in (no error)=w1309) -> (VISA resource name out=w1303:refnum<visa-resource-name>, error out=w1302:errorcluster)  [unwired: 1 out]
                      n563 = Bundle By Name(cluster=w1298, "VISA resource name out"=w1303, "error out"=w1302) -> (w1299:T1)
                    }
                    frame True {
                      n564 = global write "axxon_Gold.vi" "Feeding finished"(TRUE ("进板完成")) -> ()
                    }
                  }
                }
                frame #1 {
                  n565 = case shown="假" w1313 {
                    frame False {
                      # "马达反向"
                      n566 = call "GT_SetExtIoValue.vi"("Value"=FALSE, "index"=1, "mdl"=0) -> ()  [unwired: 3 in, 1 out]
                    }
                    frame True {
                    }
                  }
                }
                frame #2 {
                  n567 = case shown="假" w1317 {
                    frame False {
                      w1319 = 0 ("mdl")
                      # "传送马达运动"
                      n568 = call "GT_SetExtIoValue.vi"("Value"=TRUE, "index"=w1319, "mdl"=w1319) -> ()  [unwired: 3 in, 1 out]
                    }
                    frame True {
                    }
                  }
                }
                frame #3 {
                  n569 = case shown="假" w1320 {
                    tunnel: w1322 -> [w1325 _]
                    tunnel: w1321 -> [w1323 _]
                    frame False {
                      n570 = while {
                        tunnel: w1325 -> [w1343]
                        tunnel: [w1338] -> w1324
                        stop <- w1338 stop-if-true
                        n571 = call "GT_GetDi.vi"("diType in"=w1343) -> ("IOOut"=w1342:bool[])  [unwired: 2 in, 2 out]
                        n572 = global read "axxon_Gold.vi" "EmergencyStop"() -> (w1337:bool)
                        n573 = Index Array(array=w1342, index=2 ("索引")) -> (element=w1340:bool)
                        n574 = Compound Arithmetic op=OR(w1340, w1337) -> (w1338:bool)
                        n575 = Wait (ms)(milliseconds to wait=u32 1 ("等待时间（毫秒）")) -> ()  [unwired: 1 out]
                      }
                      n576 = case shown="真" w1324 {
                        tunnel: w1323 -> [_ w1326]
                        frame False {
                        }
                        frame True {
                          n577 = stacked-sequence {
                            tunnel: w1326 -> [w1327 _]
                            frame #0 {
                              n578 = case shown="真" w1327 {
                                frame False {
                                }
                                frame True {
                                n579 = global read "axxon_Gold.vi" "Discharge waiting time"() -> (w1330:dbl)
                                n580 = Multiply(x=w1330, y=1000.0) -> (x*y=w1328:dbl)
                                n581 = Wait (ms)(milliseconds to wait=w1328) -> ()  [unwired: 1 out]
                                }
                              }
                            }
                            frame #1 {
                              w1336 = 0 ("mdl")
                              # "挡板气缸"
                              # "传送马达停止"
                              n582 = call "GT_SetExtIoValue.vi"("Value"=FALSE, "index"=w1336, "mdl"=w1336) -> ("rtn_Out"=w1331:cluster{"rtn":i16, "Func":string})  [unwired: 3 in]
                              n583 = call "GT_SetExtIoValue.vi"("Value"=FALSE, "index"=6, "mdl"=0, "rtn_In"=w1331) -> ()  [unwired: 2 in, 1 out]
                            }
                          }
                        }
                      }
                    }
                    frame True {
                    }
                  }
                }
                frame #4 {
                  n584 = case shown="假" w1344 {
                    tunnel: w1345 -> [w1349 _]
                    frame False {
                      n585 = case shown="假" w1349 {
                        tunnel: 0 ("mdl") -> [w1359 _]
                        tunnel: [w1358 FALSE] -> w1347
                        tunnel: 1 ("Index") -> [w1357 _]
                        frame False {
                          n586 = global read "axxon_Gold.vi" "Cleaning waiting time"() -> (w1356:i32)
                          n587 = Tick Count (ms)() -> (millisecond timer value=w1354:u32)
                          n588 = Multiply(x=w1356, y=1000) -> (x*y=w1353:i32)
                          n589 = while {
                            tunnel: w1359 -> [w1370]
                            tunnel: [w1365] -> w1358
                            tunnel: w1357 -> [w1367]
                            tunnel: w1354 -> [w1363]
                            tunnel: w1353 -> [w1361]
                            tunnel: [w1360] -> w1352
                            stop <- w1368 stop-if-true
                            # "下位机进板信号"
                            n590 = Tick Count (ms)() -> (millisecond timer value=w1364:u32)
                            n591 = call "GT_GetExtIoBit.vi"("Index"=w1367, "mdl"=w1370) -> ("Status"=w1365:bool)  [unwired: 2 in, 1 out]
                            n592 = global read "axxon_Gold.vi" "EmergencyStop"() -> (w1366:bool)
                            n593 = Subtract(x=w1364, y=w1363) -> (x-y=w1362:u32)
                            n594 = Greater Or Equal?(x=w1362, y=w1361) -> (x >= y?=w1360:bool)
                            n595 = Compound Arithmetic op=OR(w1365, w1366, w1360) -> (w1368:bool)
                            n596 = Wait (ms)(milliseconds to wait=u32 1 ("等待时间（毫秒）")) -> ()  [unwired: 1 out]
                          }
                          n597 = global write "axxon_Gold.vi" "Waitting timeout"(w1352) -> ()
                        }
                        frame True {
                          # "离线模式"
                        }
                      }
                      n598 = case shown="真" w1347 {
                        frame False {
                        }
                        frame True {
                          w1351 = 0 ("mdl")
                          # "传送马达动"
                          n599 = call "GT_SetExtIoValue.vi"("Value"=TRUE, "index"=w1351, "mdl"=w1351) -> ()  [unwired: 3 in, 1 out]
                        }
                      }
                    }
                    frame True {
                    }
                  }
                }
                frame #5 {
                  n600 = case shown="假" w1372 {
                    tunnel: w1374 -> [w1376 _]
                    tunnel: w1373 -> [w1375 _]
                    frame False {
                      n601 = case shown="假" w1375 {
                        tunnel: w1376 -> [w1378 _]
                        frame False {
                          n602 = while {
                            tunnel: w1378 -> [w1400]
                            tunnel: [w1395] -> w1377
                            stop <- w1395 stop-if-true
                            n603 = call "GT_GetDi.vi"("diType in"=w1400) -> ("IOOut"=w1399:bool[])  [unwired: 2 in, 2 out]
                            n604 = global read "axxon_Gold.vi" "EmergencyStop"() -> (w1393:bool)
                            n605 = Index Array(array=w1399, index=2 ("索引")) -> (element=w1397:bool)
                            n606 = Not(x=w1397) -> (.not. x?=w1396:bool)
                            n607 = Wait (ms)(milliseconds to wait=u32 1 ("等待时间（毫秒）")) -> ()  [unwired: 1 out]
                            n608 = Compound Arithmetic op=OR(w1396, w1393) -> (w1395:bool)
                          }
                          n609 = case shown="真" w1377 {
                            frame False {
                            }
                            frame True {
                              w1385 = i16 2 items=["MC_Enable", "MC_Clear", "MC_Gpo"] ("doType")
                              w1392 = 0 ("mdl")
                              # "上位机进板信号"
                              # "有板信号"
                              # "挡板气缸"
                              # "传送马达停"
                              n610 = call "GT_SetExtIoValue.vi"("Value"=FALSE, "index"=w1392, "mdl"=w1392) -> ("rtn_Out"=w1381:cluster{"rtn":i16, "Func":string})  [unwired: 3 in]
                              n611 = call "GT_SetExtIoValue.vi"("Value"=FALSE, "index"=6, "mdl"=0, "rtn_In"=w1381) -> ("rtn_Out"=w1380:cluster{"rtn":i16, "Func":string})  [unwired: 2 in]
                              n612 = call "GT_SetExtIoValue.vi"("Value"=FALSE, "index"=7, "mdl"=0, "rtn_In"=w1380) -> ("rtn_Out"=w1379:cluster{"rtn":i16, "Func":string})  [unwired: 2 in]
                              n613 = call "GT_SetDoBit.vi"("Value"=TRUE, "doIndex"=i16 3, "doType"=w1385, "rtn_In"=w1379) -> ()  [unwired: 7 in, 1 out]
                            }
                          }
                        }
                        frame True {
                        }
                      }
                    }
                    frame True {
                    }
                  }
                }
              }
            }
          }
        }
        frame "左进左出" {
          w1408 = i16 4 items=["Limit_Positive", "Limit_Negative", "Alarm", "Home", "Gpi", "arrive"] ("diType in")
          # "0 到位传感器\n1 进料传感器\n2 出料传感器"
          n614 = call "GT_GetDi.vi"("diType in"=w1408) -> ("IOOut"=w1416:bool[])  [unwired: 2 in, 2 out]
          n615 = global read "axxon_Gold.vi" "Track closed"() -> (w1406:bool)
          n616 = Index Array(array=w1416, index #1=0 ("索引"), index #2=1 ("索引")) -> (element #1=w1413:bool, element #2=w1412:bool)
          n617 = case shown="假" w1413 {
            tunnel: w1412 -> [w1427 _]
            tunnel: w1405 -> [w1426 w1660]
            tunnel: w1411 -> [w1425 w1659]
            tunnel: w1410 -> [w1424 w1656]
            tunnel: w1402 -> [w1423 w1658]
            tunnel: [w1422 w1657] -> w1409
            tunnel: w1408 -> [w1421 w1655]
            tunnel: w1404 -> [w1420 _]
            tunnel: w1407 -> [w1419 _]
            tunnel: w1406 -> [w1418 w1654]
            tunnel: w1403 -> [w1417 w1653]
            tunnel: w1401 -> [_ w1652]
            frame False {
              n618 = case shown="真" w1427 {
                tunnel: w1426 -> [_ w1438]
                tunnel: w1425 -> [_ w1437]
                tunnel: w1424 -> [_ w1436]
                tunnel: w1423 -> [w1429 w1435]
                tunnel: [w1429 w1434] -> w1422
                tunnel: w1421 -> [_ w1433]
                tunnel: w1420 -> [_ w1432]
                tunnel: w1419 -> [_ w1431]
                tunnel: w1418 -> [_ w1430]
                tunnel: w1417 -> [_ _]
                frame False {
                  n619 = global write "axxon_Gold.vi" "Feeding tips"(FALSE ("进料提示")) -> ()
                }
                frame True {
                  n620 = stacked-sequence {
                    seq-local: [w1440 _] -> [_ w1450]
                    tunnel: w1438 -> [_ w1461]
                    tunnel: w1437 -> [_ w1460]
                    tunnel: w1436 -> [_ w1459]
                    tunnel: w1435 -> [_ w1458]
                    tunnel: [_ w1457] -> w1434
                    tunnel: w1433 -> [_ w1456]
                    tunnel: w1432 -> [_ w1455]
                    tunnel: w1431 -> [_ w1454]
                    tunnel: w1430 -> [_ w1453]
                    frame #0 {
                      n621 = global read "axxon_Gold.vi" "Pass board mode"() -> (w1441:bool)
                      n622 = global read "axxon_Gold.vi" "Barcode scanning"() -> (w1440:bool)
                      n623 = case shown="假" w1441 {
                        tunnel: w1440 -> [w1442 _]
                        frame False {
                          n624 = case shown="真" w1442 {
                            frame False {
                            }
                            frame True {
                              n625 = local read "Barcode"() -> (w1443:string)
                              n626 = Not Equal?(x=w1443, y="") -> (x != y?=w1444:bool)
                              n627 = case shown="真" w1444 {
                                tunnel: w1443 -> [_ w1449]
                                frame False {
                                n628 = global write "axxon_Gold.vi" "Alarminfo"("条形码为空！" ("Alarminfo")) -> ()
                                }
                                frame True {
                                n629 = call "BarCodeSelect.vi"("BarcodeIn"=w1449) -> ("ProductTyple"=w1447:string, "ProgramPath"=w1448:string)  [unwired: 1 in]
                                n630 = global write "axxon_Gold.vi" "DocumentPath"(w1448) -> ()
                                n631 = global write "axxon_Gold.vi" "BarCodeType"(w1447) -> ()
                                }
                              }
                            }
                          }
                        }
                        frame True {
                        }
                      }
                      n632 = global write "axxon_Gold.vi" "Feeding tips"(FALSE ("进料提示")) -> ()
                    }
                    frame #1 {
                      n633 = global read "axxon_Gold.vi" "Scaning completed"() -> (w1451:bool)
                      n634 = And(x=w1451, y=w1450) -> (x .and. y?=w1452:bool)
                      n635 = case shown="真" w1452 {
                        tunnel: w1461 -> [w1464 w1573]
                        tunnel: w1460 -> [w1465 w1572]
                        tunnel: w1459 -> [w1463 w1571]
                        tunnel: w1458 -> [w1470 w1570]
                        tunnel: [w1462 w1569] -> w1457
                        tunnel: w1456 -> [w1469 w1568]
                        tunnel: w1455 -> [w1466 w1567]
                        tunnel: w1454 -> [w1467 w1566]
                        tunnel: w1453 -> [w1468 w1565]
                        tunnel: w1450 -> [w1471 _]
                        frame False {
                          n636 = case shown="假" w1471 {
                            tunnel: w1470 -> [w1480 w1564]
                            tunnel: w1469 -> [w1479 _]
                            tunnel: w1468 -> [w1478 _]
                            tunnel: w1467 -> [w1477 _]
                            tunnel: w1466 -> [w1476 _]
                            tunnel: w1465 -> [w1475 _]
                            tunnel: w1464 -> [w1474 _]
                            tunnel: w1463 -> [w1473 _]
                            tunnel: [w1472 w1564] -> w1462
                            frame False {
                              n637 = stacked-sequence {
                                seq-local: [w1490 _ _ _ _ _] -> [_ _ _ w1542 _ _]
                                tunnel: w1474 -> [w1499 _ _ _ _ _]
                                tunnel: w1475 -> [w1497 _ _ _ _ _]
                                tunnel: w1473 -> [w1494 _ _ w1539 _ _]
                                tunnel: w1480 -> [w1491 _ _ _ _ _]
                                tunnel: [_ _ _ w1538 _ _] -> w1472
                                tunnel: w1479 -> [_ _ w1517 _ _ _]
                                tunnel: w1476 -> [_ _ _ w1533 _ _]
                                tunnel: w1477 -> [_ _ _ w1532 _ _]
                                tunnel: w1478 -> [w1489 _ _ _ _ _]
                                frame #0 {
                                # "马达反向"
                                # "档板气缸"
                                n638 = call "GT_SetExtIoValue.vi"("Value"=FALSE, "index"=6, "mdl"=0) -> ("rtn_Out"=w1485:cluster{"rtn":i16, "Func":string})  [unwired: 3 in]
                                n639 = call "ASCITransfer.vi"("Input"=w1499) -> ("Output"=w1498:string)
                                n640 = call "ASCITransfer.vi"("Input"=w1497) -> ("Output"=w1496:string)
                                n641 = Unbundle By Name(w1491) -> ("VISA resource name out"=w1503:refnum<visa-resource-name>, "error out"=w1502:errorcluster)
                                n642 = case shown="假" w1489 {
                                tunnel: w1485 -> [w1509 w1513]
                                tunnel: [w1504 w1513] -> w1481
                                frame False {
                                w1508 = i16 2 items=["MC_Enable", "MC_Clear", "MC_Gpo"] ("doType")
                                # "上位机进板信号"
                                # "有板信号"
                                n643 = call "GT_SetExtIoValue.vi"("Value"=FALSE, "index"=7, "mdl"=0, "rtn_In"=w1509) -> ("rtn_Out"=w1505:cluster{"rtn":i16, "Func":string})  [unwired: 2 in]
                                n644 = call "GT_SetDoBit.vi"("Value"=FALSE, "doIndex"=i16 3, "doType"=w1508, "rtn_In"=w1505) -> ("rtn_Out"=w1504:cluster{"rtn":i16, "Func":string})  [unwired: 7 in]
                                }
                                frame True {
                                }
                                }
                                n645 = Concatenate Strings("\u001f" ("字符串"), "\u0000" ("字符串"), w1498, w1496) -> (w1495:string)
                                n646 = VISA Write(VISA resource name=w1503, write buffer=w1495, error in (no error)=w1502) -> (VISA resource name out=w1493:refnum<visa-resource-name>, error out=w1492:errorcluster)  [unwired: 1 out]
                                n647 = Bundle By Name(cluster=w1494, "VISA resource name out"=w1493, "error out"=w1492) -> (w1490:T1)
                                n648 = call "GT_SetExtIoValue.vi"("Value"=FALSE, "index"=1, "mdl"=0, "rtn_In"=w1481) -> ()  [unwired: 2 in, 1 out]
                                }
                                frame #1 {
                                w1515 = 0 ("mdl")
                                # "传送马达运动"
                                n649 = call "GT_SetExtIoValue.vi"("Value"=TRUE, "index"=w1515, "mdl"=w1515) -> ()  [unwired: 3 in, 1 out]
                                }
                                frame #2 {
                                n650 = while {
                                tunnel: w1517 -> [w1530]
                                tunnel: [w1524] -> w1516
                                stop <- w1524 stop-if-true
                                # "到位检测"
                                n651 = call "GT_GetDi.vi"("diType in"=w1530) -> ("IOOut"=w1529:bool[])  [unwired: 2 in, 2 out]
                                n652 = Wait (ms)(milliseconds to wait=u32 1 ("等待时间（毫秒）")) -> ()  [unwired: 1 out]
                                n653 = global read "axxon_Gold.vi" "EmergencyStop"() -> (w1523:bool)
                                n654 = Index Array(array=w1529, index=0 ("索引")) -> (element=w1527:bool)
                                n655 = global read "axxon_Gold.vi" "Stop"() -> (w1526:bool)
                                n656 = Compound Arithmetic op=OR(w1527, w1526, w1523) -> (w1524:bool)
                                }
                                n657 = case shown="真" w1516 {
                                frame False {
                                }
                                frame True {
                                w1518 = FALSE ("Value")
                                w1522 = 0 ("mdl")
                                # "档板气缸"
                                # "传送马达停止"
                                n658 = call "GT_SetExtIoValue.vi"("Value"=w1518, "index"=6, "mdl"=0) -> ("rtn_Out"=w1519:cluster{"rtn":i16, "Func":string})  [unwired: 3 in]
                                n659 = call "GT_SetExtIoValue.vi"("Value"=w1518, "index"=w1522, "mdl"=w1522, "rtn_In"=w1519) -> ()  [unwired: 2 in, 1 out]
                                }
                                }
                                }
                                frame #3 {
                                n660 = call "ASCITransfer.vi"("Input"=w1533) -> ("Output"=w1535:string)
                                n661 = call "ASCITransfer.vi"("Input"=w1532) -> ("Output"=w1534:string)
                                n662 = Unbundle By Name(w1542) -> ("VISA resource name out"=w1544:refnum<visa-resource-name>, "error out"=w1541:errorcluster)
                                n663 = Concatenate Strings("\u001f" ("字符串"), "\u0000" ("字符串"), w1535, w1534) -> (w1531:string)
                                n664 = VISA Write(VISA resource name=w1544, write buffer=w1531, error in (no error)=w1541) -> (VISA resource name out=w1543:refnum<visa-resource-name>, error out=w1540:errorcluster)  [unwired: 1 out]
                                n665 = Bundle By Name(cluster=w1539, "VISA resource name out"=w1543, "error out"=w1540) -> (w1538:T1)
                                }
                                frame #4 {
                                w1546 = 0 ("mdl")
                                # "传送马达动"
                                n666 = call "GT_SetExtIoValue.vi"("Value"=TRUE, "index"=w1546, "mdl"=w1546) -> ()  [unwired: 3 in, 1 out]
                                }
                                frame #5 {
                                n667 = global read "axxon_Gold.vi" "Board waiting time"() -> (w1550:u32)
                                n668 = Tick Count (ms)() -> (millisecond timer value=w1551:u32)
                                n669 = Multiply(x=w1550, y=u32 1000) -> (x*y=w1548:u32)
                                n670 = while {
                                tunnel: w1551 -> [w1562]
                                tunnel: w1548 -> [w1560]
                                tunnel: [w1556] -> w1547
                                stop <- w1556 stop-if-true
                                n671 = Tick Count (ms)() -> (millisecond timer value=w1563:u32)
                                n672 = global read "axxon_Gold.vi" "EmergencyStop"() -> (w1555:bool)
                                n673 = Subtract(x=w1563, y=w1562) -> (x-y=w1561:u32)
                                n674 = global read "axxon_Gold.vi" "Stop"() -> (w1559:bool)
                                n675 = Greater Or Equal?(x=w1561, y=w1560) -> (x >= y?=w1558:bool)
                                n676 = Compound Arithmetic op=OR(w1555, w1559, w1558) -> (w1556:bool)
                                n677 = Wait (ms)(milliseconds to wait=u32 1 ("等待时间（毫秒）")) -> ()  [unwired: 1 out]
                                }
                                n678 = case shown="真" w1547 {
                                frame False {
                                }
                                frame True {
                                w1554 = 0 ("mdl")
                                # "马达运动停止"
                                n679 = global write "axxon_Gold.vi" "Feeding finished"(TRUE ("进板完成")) -> ()
                                n680 = call "GT_SetExtIoValue.vi"("Value"=FALSE, "index"=w1554, "mdl"=w1554) -> ()  [unwired: 3 in, 1 out]
                                }
                                }
                                }
                              }
                            }
                            frame True {
                            }
                          }
                        }
                        frame True {
                          n681 = stacked-sequence {
                            seq-local: [w1583 _ _ _ _ _] -> [_ _ _ w1631 _ _]
                            tunnel: w1573 -> [w1592 _ _ _ _ _]
                            tunnel: w1572 -> [w1590 _ _ _ _ _]
                            tunnel: w1571 -> [w1587 _ _ w1628 _ _]
                            tunnel: w1570 -> [w1584 _ _ _ _ _]
                            tunnel: [_ _ _ w1627 _ _] -> w1569
                            tunnel: w1568 -> [_ _ w1610 _ _ _]
                            tunnel: w1567 -> [_ _ _ w1622 _ _]
                            tunnel: w1566 -> [_ _ _ w1621 _ _]
                            tunnel: w1565 -> [w1582 _ _ _ _ _]
                            frame #0 {
                              # "档板气缸"
                              # "马达反向"
                              n682 = call "GT_SetExtIoValue.vi"("Value"=FALSE, "index"=1, "mdl"=0) -> ("rtn_Out"=w1578:cluster{"rtn":i16, "Func":string})  [unwired: 3 in]
                              n683 = call "ASCITransfer.vi"("Input"=w1592) -> ("Output"=w1591:string)
                              n684 = call "ASCITransfer.vi"("Input"=w1590) -> ("Output"=w1589:string)
                              n685 = Unbundle By Name(w1584) -> ("VISA resource name out"=w1596:refnum<visa-resource-name>, "error out"=w1595:errorcluster)
                              n686 = case shown="假" w1582 {
                                tunnel: w1578 -> [w1599 w1606]
                                tunnel: [w1597 w1606] -> w1574
                                frame False {
                                w1605 = i16 2 items=["MC_Enable", "MC_Clear", "MC_Gpo"] ("doType")
                                # "有板信号"
                                # "上位机进板信号"
                                n687 = call "GT_SetDoBit.vi"("Value"=FALSE, "doIndex"=i16 3, "doType"=w1605, "rtn_In"=w1599) -> ("rtn_Out"=w1598:cluster{"rtn":i16, "Func":string})  [unwired: 7 in]
                                n688 = call "GT_SetExtIoValue.vi"("Value"=FALSE, "index"=7, "mdl"=0, "rtn_In"=w1598) -> ("rtn_Out"=w1597:cluster{"rtn":i16, "Func":string})  [unwired: 2 in]
                                }
                                frame True {
                                }
                              }
                              n689 = Concatenate Strings("\u001f" ("字符串"), "\u0000" ("字符串"), w1591, w1589) -> (w1588:string)
                              n690 = VISA Write(VISA resource name=w1596, write buffer=w1588, error in (no error)=w1595) -> (VISA resource name out=w1586:refnum<visa-resource-name>, error out=w1585:errorcluster)  [unwired: 1 out]
                              n691 = Bundle By Name(cluster=w1587, "VISA resource name out"=w1586, "error out"=w1585) -> (w1583:T1)
                              n692 = call "GT_SetExtIoValue.vi"("Value"=FALSE, "index"=6, "mdl"=0, "rtn_In"=w1574) -> ()  [unwired: 2 in, 1 out]
                            }
                            frame #1 {
                              w1608 = 0 ("mdl")
                              # "传送马达运动"
                              n693 = call "GT_SetExtIoValue.vi"("Value"=TRUE, "index"=w1608, "mdl"=w1608) -> ()  [unwired: 3 in, 1 out]
                            }
                            frame #2 {
                              n694 = while {
                                tunnel: w1610 -> [w1619]
                                tunnel: [w1614] -> w1609
                                stop <- w1614 stop-if-true
                                # "到位检测"
                                n695 = call "GT_GetDi.vi"("diType in"=w1619) -> ("IOOut"=w1618:bool[])  [unwired: 2 in, 2 out]
                                n696 = Wait (ms)(milliseconds to wait=u32 1 ("等待时间（毫秒）")) -> ()  [unwired: 1 out]
                                n697 = global read "axxon_Gold.vi" "EmergencyStop"() -> (w1613:bool)
                                n698 = Index Array(array=w1618, index=0 ("索引")) -> (element=w1616:bool)
                                n699 = Compound Arithmetic op=OR(w1616, w1613) -> (w1614:bool)
                              }
                              n700 = case shown="真" w1609 {
                                frame False {
                                }
                                frame True {
                                w1612 = 0 ("mdl")
                                # "传送马达停止"
                                n701 = call "GT_SetExtIoValue.vi"("Value"=FALSE, "index"=w1612, "mdl"=w1612) -> ()  [unwired: 3 in, 1 out]
                                }
                              }
                            }
                            frame #3 {
                              n702 = call "ASCITransfer.vi"("Input"=w1622) -> ("Output"=w1624:string)
                              n703 = call "ASCITransfer.vi"("Input"=w1621) -> ("Output"=w1623:string)
                              n704 = Unbundle By Name(w1631) -> ("VISA resource name out"=w1633:refnum<visa-resource-name>, "error out"=w1630:errorcluster)
                              n705 = Concatenate Strings("\u001f" ("字符串"), "\u0000" ("字符串"), w1624, w1623) -> (w1620:string)
                              n706 = VISA Write(VISA resource name=w1633, write buffer=w1620, error in (no error)=w1630) -> (VISA resource name out=w1632:refnum<visa-resource-name>, error out=w1629:errorcluster)  [unwired: 1 out]
                              n707 = Bundle By Name(cluster=w1628, "VISA resource name out"=w1632, "error out"=w1629) -> (w1627:T1)
                            }
                            frame #4 {
                              w1635 = 0 ("mdl")
                              # "传送马达动"
                              n708 = call "GT_SetExtIoValue.vi"("Value"=TRUE, "index"=w1635, "mdl"=w1635) -> ()  [unwired: 3 in, 1 out]
                            }
                            frame #5 {
                              n709 = global read "axxon_Gold.vi" "Board waiting time"() -> (w1639:u32)
                              n710 = Tick Count (ms)() -> (millisecond timer value=w1640:u32)
                              n711 = Multiply(x=w1639, y=u32 1000) -> (x*y=w1637:u32)
                              n712 = while {
                                tunnel: w1640 -> [w1650]
                                tunnel: w1637 -> [w1648]
                                tunnel: [w1645] -> w1636
                                stop <- w1645 stop-if-true
                                n713 = Tick Count (ms)() -> (millisecond timer value=w1651:u32)
                                n714 = global read "axxon_Gold.vi" "EmergencyStop"() -> (w1644:bool)
                                n715 = Subtract(x=w1651, y=w1650) -> (x-y=w1649:u32)
                                n716 = Greater Or Equal?(x=w1649, y=w1648) -> (x >= y?=w1647:bool)
                                n717 = Compound Arithmetic op=OR(w1644, w1647) -> (w1645:bool)
                                n718 = Wait (ms)(milliseconds to wait=u32 1 ("等待时间（毫秒）")) -> ()  [unwired: 1 out]
                              }
                              n719 = case shown="真" w1636 {
                                frame False {
                                }
                                frame True {
                                w1643 = 0 ("mdl")
                                # "马达运动停止"
                                n720 = global write "axxon_Gold.vi" "Feeding finished"(TRUE ("进板完成")) -> ()
                                n721 = call "GT_SetExtIoValue.vi"("Value"=FALSE, "index"=w1643, "mdl"=w1643) -> ()  [unwired: 3 in, 1 out]
                                }
                              }
                            }
                          }
                        }
                      }
                    }
                  }
                }
              }
            }
            frame True {
              n722 = stacked-sequence {
                seq-local: [w1662 _ _ _ _ _] -> [_ w1690 w1694 w1697 w1721 w1749]
                tunnel: w1660 -> [_ _ _ _ _ _]
                tunnel: w1659 -> [w1667 _ _ _ _ _]
                tunnel: w1658 -> [w1666 _ _ _ _ _]
                tunnel: [w1665 _ _ _ _ _] -> w1657
                tunnel: w1656 -> [w1664 _ _ _ _ _]
                tunnel: w1655 -> [_ _ _ w1699 _ w1751]
                tunnel: w1654 -> [_ _ _ w1698 w1722 w1750]
                tunnel: w1653 -> [w1663 _ _ _ _ _]
                tunnel: w1652 -> [w1661 _ _ _ _ _]
                frame #0 {
                  n723 = case shown="真" w1661 {
                    tunnel: [TRUE ("T button?") w1673] -> w1662
                    frame False {
                    }
                    frame True {
                      n724 = global write "axxon_Gold.vi" "Feeding tips"(FALSE ("进料提示")) -> ()
                      n725 = Two Button Dialog(message="轨道上有板，是否继续涂！" ("消息"), 1:"取消" ("F按钮名称（“取消”）"), 2:"确定" ("T按钮名称（“确定”）")) -> (T button?=w1673:bool)
                    }
                  }
                  n726 = case shown="真" w1662 {
                    tunnel: w1667 -> [w1678 _]
                    tunnel: w1666 -> [w1677 w1689]
                    tunnel: [w1676 w1689] -> w1665
                    tunnel: w1664 -> [w1675 _]
                    tunnel: w1663 -> [w1674 _]
                    frame False {
                      n727 = call "ASCITransfer.vi"("Input"=w1674) -> ("Output"=w1683:string)
                      n728 = call "ASCITransfer.vi"("Input"=w1678) -> ("Output"=w1682:string)
                      n729 = Unbundle By Name(w1677) -> ("VISA resource name out"=w1687:refnum<visa-resource-name>, "error out"=w1686:errorcluster)
                      n730 = Concatenate Strings("\u001f" ("字符串"), "\u0000" ("字符串"), w1683, w1682) -> (w1681:string)
                      n731 = VISA Write(VISA resource name=w1687, write buffer=w1681, error in (no error)=w1686) -> (VISA resource name out=w1680:refnum<visa-resource-name>, error out=w1679:errorcluster)  [unwired: 1 out]
                      n732 = Bundle By Name(cluster=w1675, "VISA resource name out"=w1680, "error out"=w1679) -> (w1676:T1)
                    }
                    frame True {
                      n733 = global write "axxon_Gold.vi" "Feeding finished"(TRUE ("进板完成")) -> ()
                    }
                  }
                }
                frame #1 {
                  n734 = case shown="假" w1690 {
                    frame False {
                      # "电机反转"
                      n735 = call "GT_SetExtIoValue.vi"("Value"=TRUE, "index"=1, "mdl"=0) -> ()  [unwired: 3 in, 1 out]
                    }
                    frame True {
                    }
                  }
                }
                frame #2 {
                  n736 = case shown="假" w1694 {
                    frame False {
                      w1696 = 0 ("mdl")
                      # "传送马达运动"
                      n737 = call "GT_SetExtIoValue.vi"("Value"=TRUE, "index"=w1696, "mdl"=w1696) -> ()  [unwired: 3 in, 1 out]
                    }
                    frame True {
                    }
                  }
                }
                frame #3 {
                  n738 = case shown="假" w1697 {
                    tunnel: w1699 -> [w1702 _]
                    tunnel: w1698 -> [w1700 _]
                    frame False {
                      n739 = while {
                        tunnel: w1702 -> [w1720]
                        tunnel: [w1715] -> w1701
                        stop <- w1715 stop-if-true
                        n740 = call "GT_GetDi.vi"("diType in"=w1720) -> ("IOOut"=w1719:bool[])  [unwired: 2 in, 2 out]
                        n741 = global read "axxon_Gold.vi" "EmergencyStop"() -> (w1714:bool)
                        n742 = Index Array(array=w1719, index=1 ("索引")) -> (element=w1717:bool)
                        n743 = Compound Arithmetic op=OR(w1717, w1714) -> (w1715:bool)
                        n744 = Wait (ms)(milliseconds to wait=u32 1 ("等待时间（毫秒）")) -> ()  [unwired: 1 out]
                      }
                      n745 = case shown="真" w1701 {
                        tunnel: w1700 -> [_ w1703]
                        frame False {
                        }
                        frame True {
                          n746 = stacked-sequence {
                            tunnel: w1703 -> [w1704 _]
                            frame #0 {
                              n747 = case shown="真" w1704 {
                                frame False {
                                }
                                frame True {
                                n748 = global read "axxon_Gold.vi" "Discharge waiting time"() -> (w1707:dbl)
                                n749 = Multiply(x=w1707, y=1000.0) -> (x*y=w1705:dbl)
                                n750 = Wait (ms)(milliseconds to wait=w1705) -> ()  [unwired: 1 out]
                                }
                              }
                            }
                            frame #1 {
                              w1713 = 0 ("mdl")
                              # "挡板气缸"
                              # "传送马达停止"
                              n751 = call "GT_SetExtIoValue.vi"("Value"=FALSE, "index"=w1713, "mdl"=w1713) -> ("rtn_Out"=w1708:cluster{"rtn":i16, "Func":string})  [unwired: 3 in]
                              n752 = call "GT_SetExtIoValue.vi"("Value"=FALSE, "index"=6, "mdl"=0, "rtn_In"=w1708) -> ()  [unwired: 2 in, 1 out]
                            }
                          }
                        }
                      }
                    }
                    frame True {
                    }
                  }
                }
                frame #4 {
                  n753 = case shown="假" w1721 {
                    tunnel: w1722 -> [w1726 _]
                    frame False {
                      n754 = case shown="假" w1726 {
                        tunnel: 0 ("mdl") -> [w1736 _]
                        tunnel: [w1735 FALSE] -> w1724
                        tunnel: 1 ("Index") -> [w1734 _]
                        frame False {
                          n755 = Tick Count (ms)() -> (millisecond timer value=w1731:u32)
                          n756 = global read "axxon_Gold.vi" "Cleaning waiting time"() -> (w1733:i32)
                          n757 = Multiply(x=w1733, y=1000) -> (x*y=w1730:i32)
                          n758 = while {
                            tunnel: w1736 -> [w1747]
                            tunnel: [w1742] -> w1735
                            tunnel: w1734 -> [w1744]
                            tunnel: w1731 -> [w1740]
                            tunnel: w1730 -> [w1738]
                            tunnel: [w1737] -> w1729
                            stop <- w1745 stop-if-true
                            # "下位机进板信号"
                            n759 = Tick Count (ms)() -> (millisecond timer value=w1741:u32)
                            n760 = call "GT_GetExtIoBit.vi"("Index"=w1744, "mdl"=w1747) -> ("Status"=w1742:bool)  [unwired: 2 in, 1 out]
                            n761 = global read "axxon_Gold.vi" "EmergencyStop"() -> (w1743:bool)
                            n762 = Subtract(x=w1741, y=w1740) -> (x-y=w1739:u32)
                            n763 = Greater Or Equal?(x=w1739, y=w1738) -> (x >= y?=w1737:bool)
                            n764 = Compound Arithmetic op=OR(w1742, w1743, w1737) -> (w1745:bool)
                            n765 = Wait (ms)(milliseconds to wait=u32 1 ("等待时间（毫秒）")) -> ()  [unwired: 1 out]
                          }
                          n766 = global write "axxon_Gold.vi" "Waitting timeout"(w1729) -> ()
                        }
                        frame True {
                          # "离线模式"
                        }
                      }
                      n767 = case shown="真" w1724 {
                        frame False {
                        }
                        frame True {
                          w1728 = 0 ("mdl")
                          # "传送马达动"
                          n768 = call "GT_SetExtIoValue.vi"("Value"=TRUE, "index"=w1728, "mdl"=w1728) -> ()  [unwired: 3 in, 1 out]
                        }
                      }
                    }
                    frame True {
                    }
                  }
                }
                frame #5 {
                  n769 = case shown="假" w1749 {
                    tunnel: w1751 -> [w1753 _]
                    tunnel: w1750 -> [w1752 _]
                    frame False {
                      n770 = case shown="假" w1752 {
                        tunnel: w1753 -> [w1755 _]
                        frame False {
                          n771 = while {
                            tunnel: w1755 -> [w1777]
                            tunnel: [w1772] -> w1754
                            stop <- w1772 stop-if-true
                            n772 = call "GT_GetDi.vi"("diType in"=w1777) -> ("IOOut"=w1776:bool[])  [unwired: 2 in, 2 out]
                            n773 = global read "axxon_Gold.vi" "EmergencyStop"() -> (w1770:bool)
                            n774 = Index Array(array=w1776, index=1 ("索引")) -> (element=w1774:bool)
                            n775 = Not(x=w1774) -> (.not. x?=w1773:bool)
                            n776 = Wait (ms)(milliseconds to wait=u32 1 ("等待时间（毫秒）")) -> ()  [unwired: 1 out]
                            n777 = Compound Arithmetic op=OR(w1773, w1770) -> (w1772:bool)
                          }
                          n778 = case shown="真" w1754 {
                            frame False {
                            }
                            frame True {
                              w1762 = i16 2 items=["MC_Enable", "MC_Clear", "MC_Gpo"] ("doType")
                              w1769 = 0 ("mdl")
                              # "上位机进板信号"
                              # "有板信号"
                              # "挡板气缸"
                              # "传送马达停"
                              n779 = call "GT_SetExtIoValue.vi"("Value"=FALSE, "index"=w1769, "mdl"=w1769) -> ("rtn_Out"=w1758:cluster{"rtn":i16, "Func":string})  [unwired: 3 in]
                              n780 = call "GT_SetExtIoValue.vi"("Value"=FALSE, "index"=6, "mdl"=0, "rtn_In"=w1758) -> ("rtn_Out"=w1757:cluster{"rtn":i16, "Func":string})  [unwired: 2 in]
                              n781 = call "GT_SetExtIoValue.vi"("Value"=FALSE, "index"=7, "mdl"=0, "rtn_In"=w1757) -> ("rtn_Out"=w1756:cluster{"rtn":i16, "Func":string})  [unwired: 2 in]
                              n782 = call "GT_SetDoBit.vi"("Value"=TRUE, "doIndex"=i16 3, "doType"=w1762, "rtn_In"=w1756) -> ()  [unwired: 7 in, 1 out]
                            }
                          }
                        }
                        frame True {
                        }
                      }
                    }
                    frame True {
                    }
                  }
                }
              }
            }
          }
        }
      }
      n783 = global write "axxon_Gold.vi" "Com2"(w16) -> ()
    }
    frame True {
    }
  }
